vi "BRig_RT_start_v1,06.vi"() -> ()   [LabVIEW 2014]
uses:
  <vilib>/Platform/TimedLoop/XDataNode/XDataNode.xnode
  <vilib>/Platform/TimedLoop/XDataNode/nitl_modes.ctl
  <vilib>/Platform/TimedLoop/XDataNode/XDNodeRunTimeDep.lvlib
  <vilib>/Platform/TimedLoop/XDataNode/wakeup.ctl
  <vilib>/Platform/TimedLoop/XDataNode/timing_clust.ctl
  <vilib>/rvi/interface/nirviReadWriteControl/nirviReadWriteControl.xnode
  <vilib>/rvi/interface/Simulation/niFpgaSimulationCallBeginRW.vi
  <vilib>/rvi/errors/niLvFpgaAdjustHostInterfaceError.vi
  <vilib>/rvi/interface/nirviCloseFPGA/nirviCloseFPGA.xnode
  <vilib>/myRIO/Instrument Drivers/Utilities/Utilities.lvlib
  <vilib>/rvi/interface/nirviOpenFPGA/nirviOpenFPGA.xnode
  myRIO_BRig_RT__Case_Exp_stateList.ctl
  myRIO_BRig_RT__Case_NonExp_stateList.ctl
  <vilib>/WebDAVClient/Advanced/SessionHandle.ctl
  <vilib>/WebDAVClient/NI_WebDAV.lvlib
  <vilib>/Utility/file.llb/Read From Spreadsheet File (I64).vi
  <vilib>/Utility/file.llb/Write To Spreadsheet File (DBL).vi
  BRig_FPGA_v3,91__build.lvbitx
  BRig_FPGA_v3,91.vi
  <vilib>/FPGAPlugInAG/Dynamic/niLvFpga_Close_Dynamic.vi
panel:
  out "FreeReward_c_R":u16
  out "FreeReward_c_L":u16
  in  "Laser2_LED":bool
  in  "Laser1_LED":bool
  in  "lick_Rising(F)_or_Falling(T)":bool
  out "T_ExpRun_min":dbl
  out "stop_TimedLoop":bool
  out "BTPR_avg_R":dbl
  out "T2R_avg_R":dbl
  out "BTPR_avg_L":dbl
  out "T2R_avg_L":dbl
  out "BTPR_block":u16
  out "T2R_block":u16
  in  "comm_WebDAV_connect":bool
  in  "I_sendData":bool
  in  "comm_TCP_connect":bool
  out "nRewards_total":u16 caption="# Rewards in Current Block"
  out "BUR_target":u16 caption="Target Trials Per Block"
  in  "input_Threshold_reset":bool
  out "nTrial":u16
  out "allReward_R":bool
  out "allReward_L":bool
  out "Threshold":bool
  out "tLoop":dbl format="%#_2g"
  out "L_Power_l2":dbl
  out "comm_TCP":bool
  in  "get_countPerMS":bool
  out "SolenoidReward":bool
  out "L_Power_l1":dbl caption="LaserPower"
  in  "Recording":bool
  out "FPGA_count2ms":dbl=159.0
  out "error out":errorcluster
  out "cSpout":enum16{"Left", "Right"}(ring) caption="Left or Right Spout"
  out "A4":u32 caption="LickCounter_Right"
  out "A2":u32 caption="LickCounter_Left"
  out "nRewards_Right":u16 caption="# Rewards Total (Right)"
  out "nRewards_Left":u16 caption="# Rewards Total (Left)"
  out "nRewards_cur":u16 caption="# Rewards in Current Block"
  out "TpB_target":u16 caption="Target Trials Per Block"
  out "cState_NonExp":T1 caption="WarmUp State"
  out "iBlock":u16 caption="Current Block"
  out "cState":T2 caption="Experimental State"
  out "iTrial":u16 caption="Current Trial"
  in  "Data Set Prefix":string="Exp1_TM2"
  out "comm_WebDAV":bool
  in  "Host Password":string="sabalab"
  in  "Host UserName":string="Test2"
  in  "STOP_abort":bool caption="Stop LabView\n(Stops myRio and FPGA)"
  in  "STOP_endBlock":bool caption="Stop Experiment\n@ End of Block"
  in  "STOP_endTrial":bool caption="Stop Experiment\n@ End of Trial"
  in  "START":bool caption="Start Experiment"
  # "Experimental Run"
  # "Recording Rig"
  # "FPGA Conversion\n[counts per ms]"
  # "RealTime Cycle\nShould be <5ms"
  # "STOP experiment at"
  # "Exp Run Time"
  # "Reset"
  # "min"
  # "Communication with Host"
  # "Test AnalogInput Plotting"
  # "Lick Counter"
  # "Give Water?\n(Reward)"
  # "Experimental State"
  # "Left/Right"
  # "AI0               AI1"
  # "Left           Right"
  # "Direction\n(NonSpecific Licking)"
  # "Block Target"
  # "# Blocks"
  # "L          R"
  # "# Trials"
  # "# Rewards"
  # "Bad Trials\nPost Reward"
  # "Trials 2 Reward"
  # "Block"
  # "# Trials"
  # "# Rewards"
  # "Current\nBlock"
  # "WarmUp State"
  # "avg L"
  # "Total"
  # "# Rewards"
  # "# Trials"
  # "avg R"
  # "Laser Power [V]"
  # "Left           Right"
  # "FreeRewards"
  # "Laser1"
  # "Laser2"
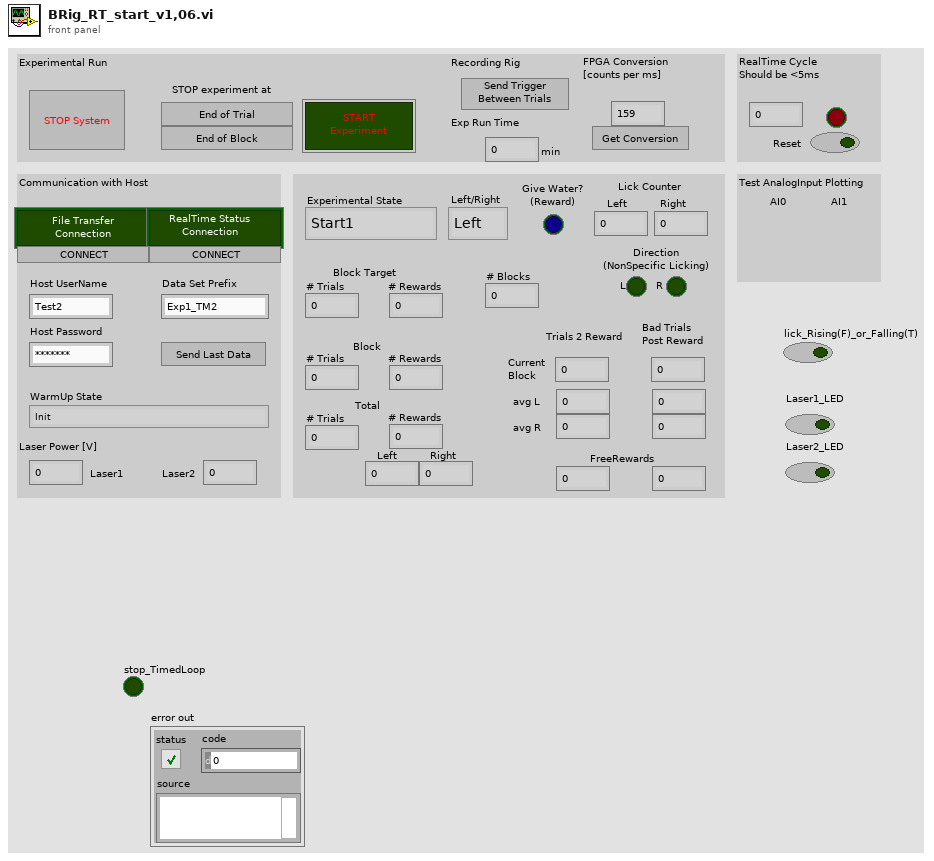
[diagram p1: front panel]
types:
  T1 = typedef "myRIO_BRig_RT__Case_NonExp_stateList.ctl" = enum16{"Init", "UploadSettings_pre", "UploadSettings_Read_dataExp", "UploadSettings_dataExp_1", "UploadSettings_dataExp_2", "UploadSettings_Read_dataLC", "UploadSettings_dataLC_1", "UploadSettings_dataLC_2", "UploadSettings_dataLC_3", "UploadSettings_dataLC_4", "UploadSettings_Read_dataMTrig", "UploadSettings_dataMTrig_1", "UploadSettings_post", "Idle_pre", "IdleEmpty", "IdleEmpty2", "IdleEmpty3", "IdleEmpty4", "Idle", "Idle_2", "Idle_3", "Idle_4", "Idle_5", "Idle_6", "Idle_post", "Cue_pre__pre", "Cue_pre", "Cue", "Cue_LED", "Cue_post", "RewardCalibration_pre", "RewardCalibration", "DispenseWater_pre__pre", "DispenseWater_pre", "DispenseWater", "DispenseWater_post", "TestConnection", "SendData", "Get_FPGA_count_per_ms", "End", "commTCP_connect"}
  T2 = typedef "myRIO_BRig_RT__Case_Exp_stateList.ctl" = enum16{"Start1", "Start2", "Start3", "saveSettings1", "saveSettings2", "saveSettings3", "saveSettings4", "saveSettings_LC_ENL_l1", "saveSettings_LC_ENL_l2", "saveSettings_LC_Cue_l1", "saveSettings_LC_Cue_l2", "saveSettings6_LC_l1_Other", "SaveSettings6_LC_l2_Other", "setSettings_Audio", "setSettings_Laser", "initBlock_pre", "initBlock", "initBlock2", "initBlock_post", "initTrial_pre", "initTrial", "initTrial2", "initTrial3", "initTrial4", "initTrial_LC_ENL1", "initTrial_LC_Cue1", "initTrial_LC_Cue1_2", "initTrial_LC_Sel", "initTrial_post", "ENL1_pre", "ENL1", "ENL1_post", "ENL1Penalty_pre", "ENL1Penalty", "ENL2_pre", "ENL2", "ENL2Penalty_pre", "ENL2Penalty", "Cue1_pre", "Cue1", "Cue1_post", "Cue1Penalty_pre", "Cue1Penalty", "Cue2_pre", "Cue2", "Cue2Penalty_pre", "Cue2Penalty", "Selection_pre", "Selection", "Select_post", "SelectReward_pre", "SelectReward", "SelectRewardPost_pre", "SelectRewardPost", "SelectWrong_pre", "SelectWrong", "SelectWrong_post", "SelectTimeout_pre", "SelectTimeout", "SelectTimeout_post", "endTrial_pre", "endTrial1", "endTrial2", "endTrial3", "endTrial_post", "endBlock_pre", "endBlock", "endBlock_post", "endExp", "commConnect", "commUpload_pre", "commUpload_dataBlock", "commUpload_dataCurrent", "commUpload_dataExp", "commUpload_dataLC", "commUpload_dataTrial", "commUpload_post", "saveData_pre", "saveData_dataBlock", "saveData_dataCurrent", "saveData_dataExp", "saveData_dataLC", "saveData_dataTrial", "saveData_post", "empty_endBlock1", "empty_endBlock2", "empty_endTrial1", "empty_endTrial2", "empty_endTrial3", "empty_endTrial4", "empty_endTrial5", "dummyState", "dummyState_endBlock", "FreeReward_pre", "FreeReward", "FreeRewardPost_pre", "FreeRewardPost"}
  T3 = enum8{"Enabled", "Disabled", "Disabled and Grayed Out"}
  T4 = typedef "NI_WebDAV.lvlib/SessionHandle.ctl" = refnum<k1>
  T5 = typedef "XDNodeRunTimeDep.lvlib/timing_clust.ctl" = cluster{"Expected End [f-1]":u64, "Actual End [f-1]":u64, "Finished Late? [f-1]":bool, "Expected End [i-1]":u64, "Actual End [i-1]":u64, "Finished Late? [i-1]":bool, "Expected Start [i]":u64, "Actual Start [i]":u64, "Expected Start [f]":u64, "Actual Start [f]":u64, "Source Name":string, "Structure Name":string, "Period":i64, "Deadline":i64, "Offset":i64, "Start":i64, "Priority":i32, "Timeout":i32, "Mode":T6, "Wakeup Reason":T7, "Error":errorcluster, "Source Type":string, "Secondary Source Type":string, "Global End Time":u64, "Global Start Time":u64, "Frame Duration":u64, "Iteration Duration":u64, "Assigned CPU":i32, "I/O Scan Engine Mode":u32}
  T6 = typedef "XDNodeRunTimeDep.lvlib/nitl_modes.ctl" = enum32{"No Change", "Process missed periods, maintain original phase", "Discard missed periods, maintain original phase", "Process missed periods, ignore original phase", "Discard missed periods, ignore original phase"}
  T7 = typedef "XDNodeRunTimeDep.lvlib/wakeup.ctl" = enum32{"Normal", "Aborted", "Asynchronous wakeup", "Timing source error", "Timed loop error", "Timeout"}
  T8 = cluster{"read mode":enum16{"polling", "blocking"}, "write mode":enum16{"polling", "blocking"}}
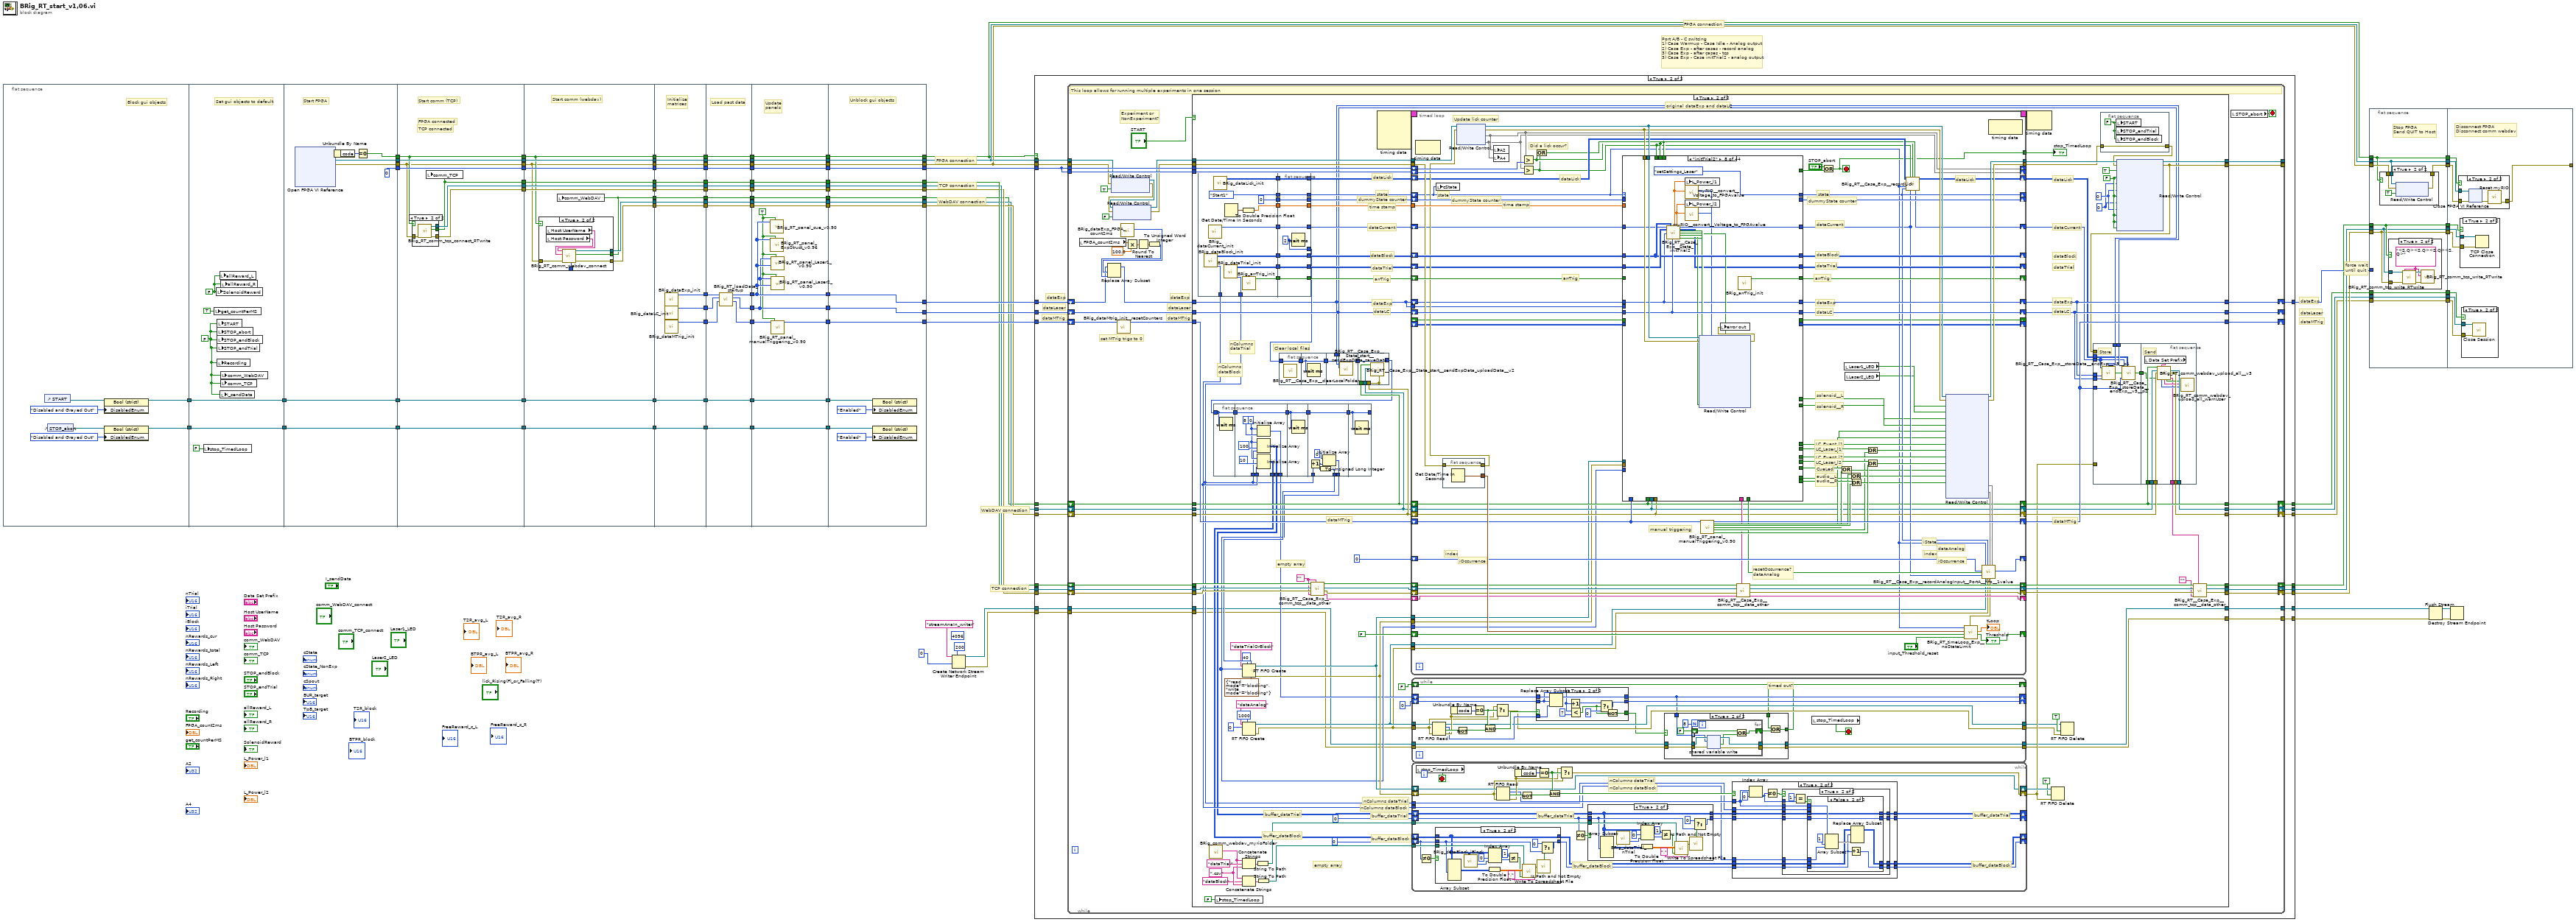
[diagram p0: block diagram]
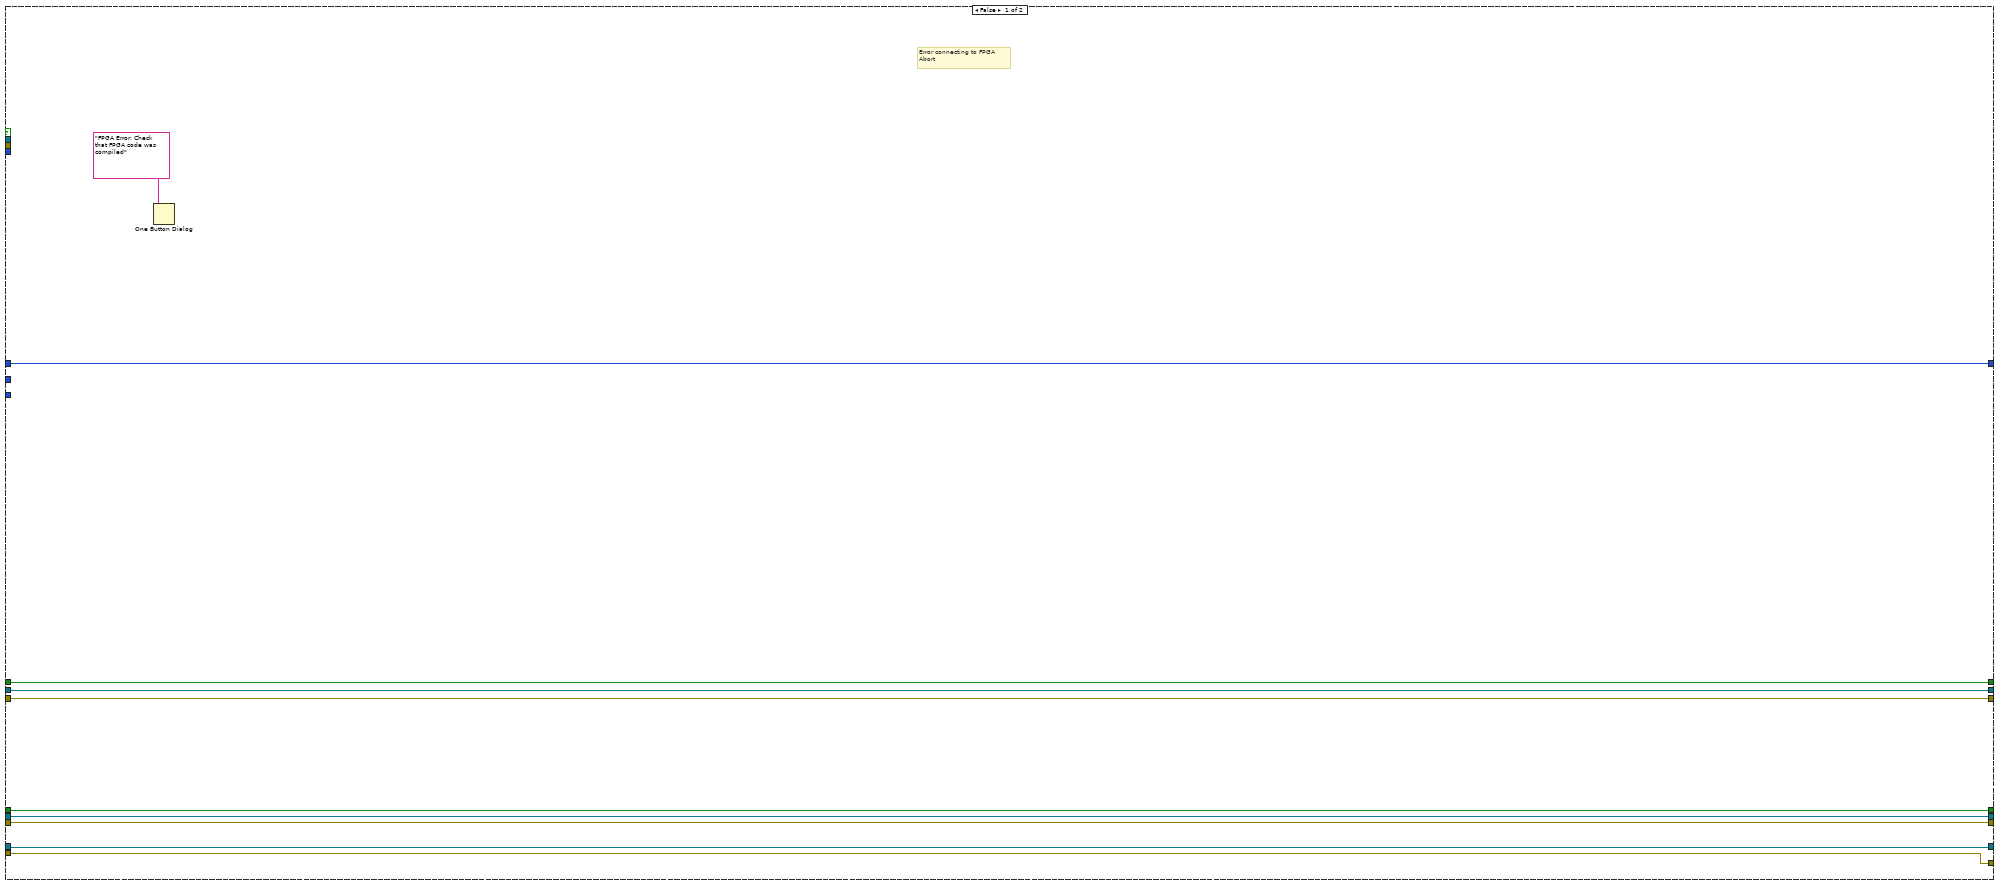
[diagram p2: hidden frame]
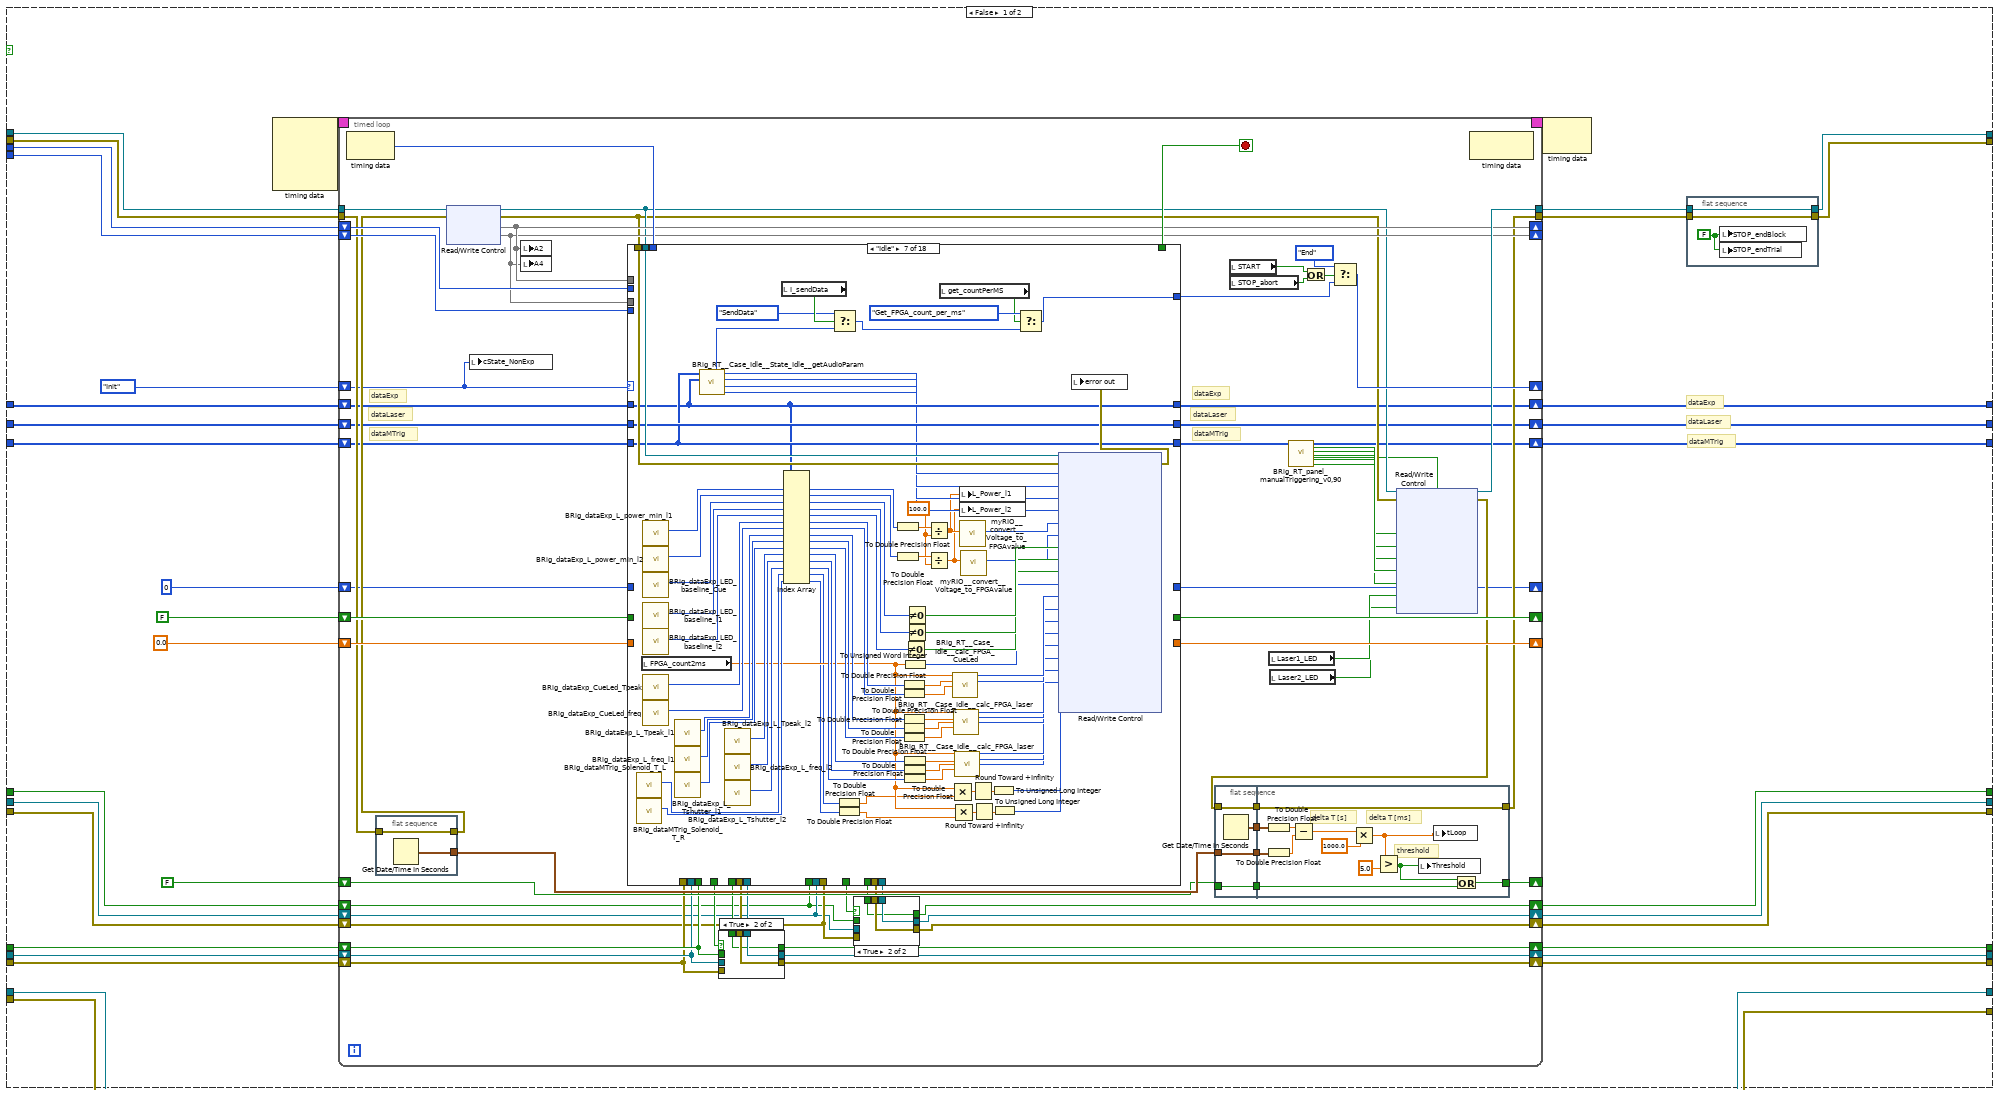
[diagram p3: hidden frame]
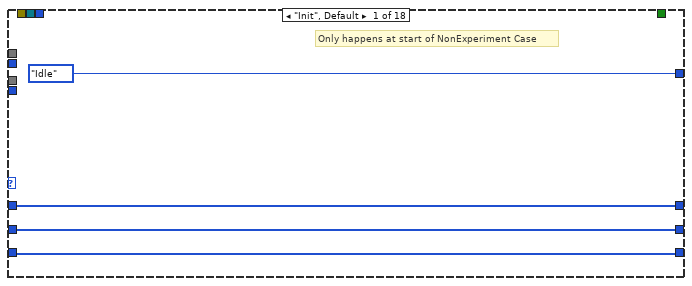
[diagram p6: hidden frame]
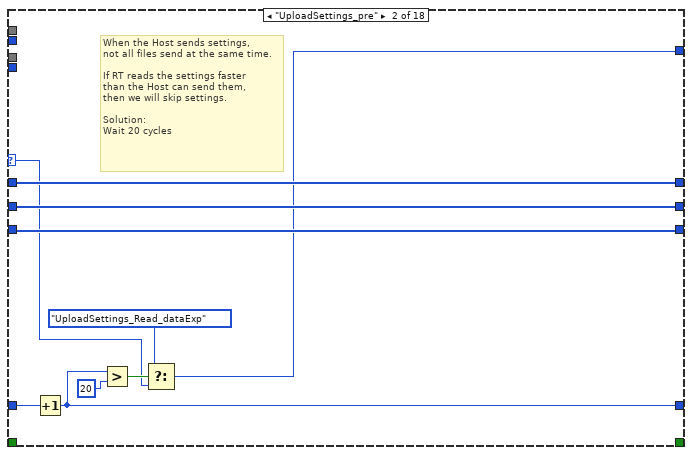
[diagram p7: hidden frame]
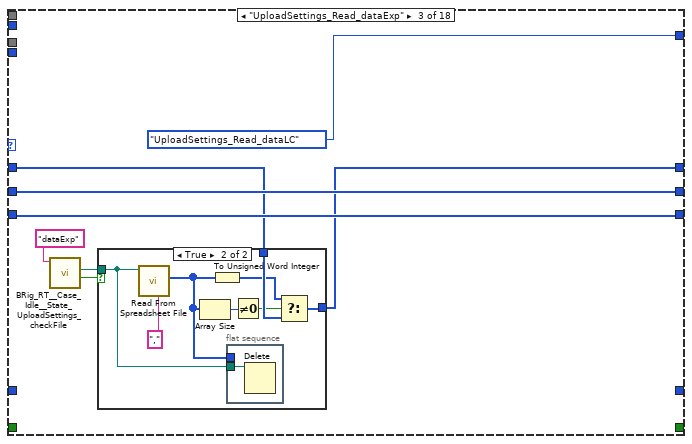
[diagram p8: hidden frame]
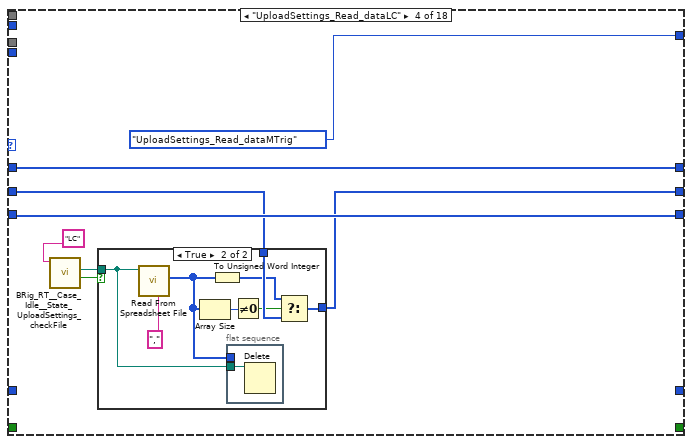
[diagram p10: hidden frame]
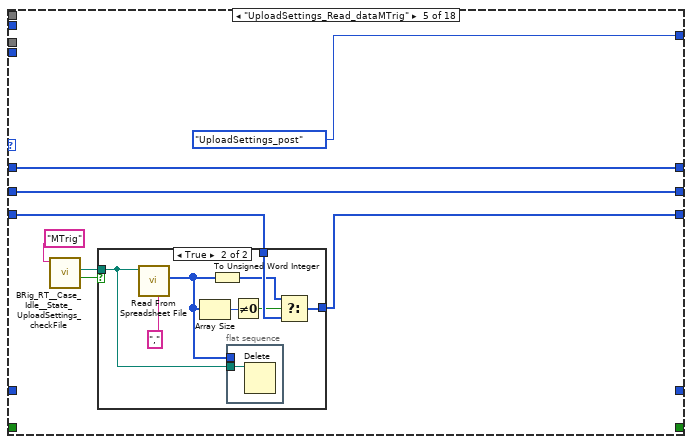
[diagram p12: hidden frame]
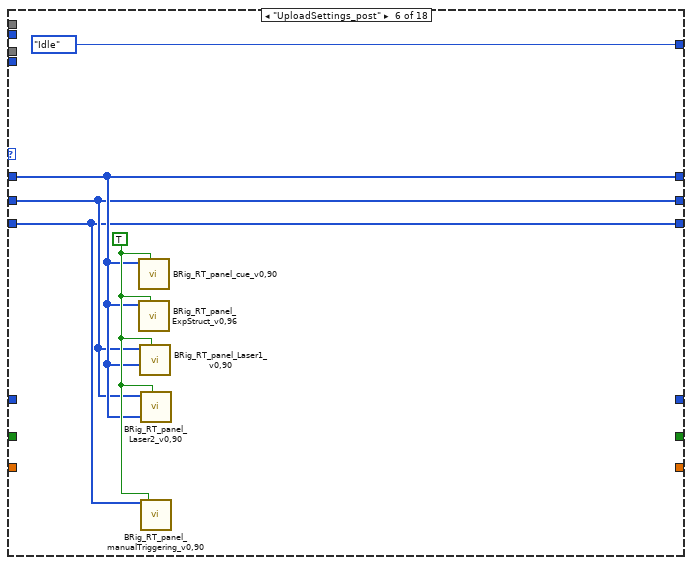
[diagram p14: hidden frame]
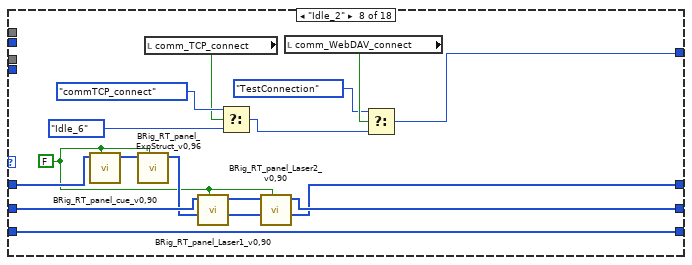
[diagram p15: hidden frame]
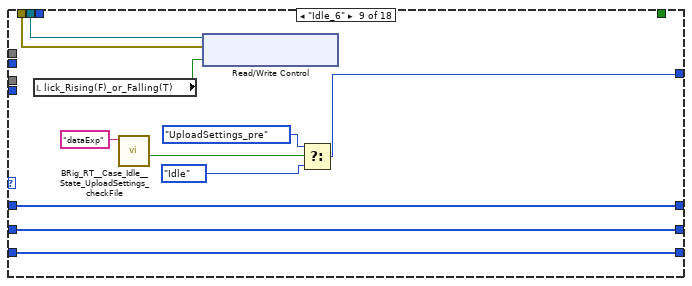
[diagram p16: hidden frame]
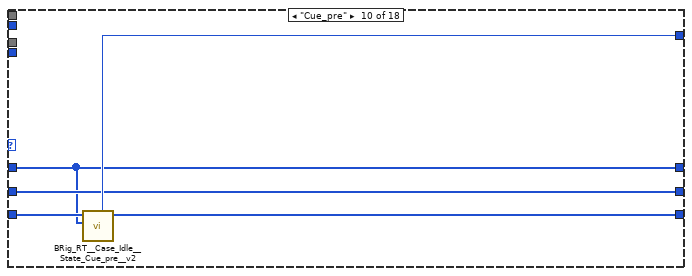
[diagram p17: hidden frame]
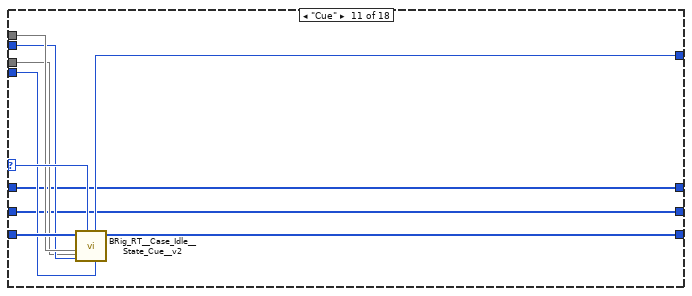
[diagram p18: hidden frame]
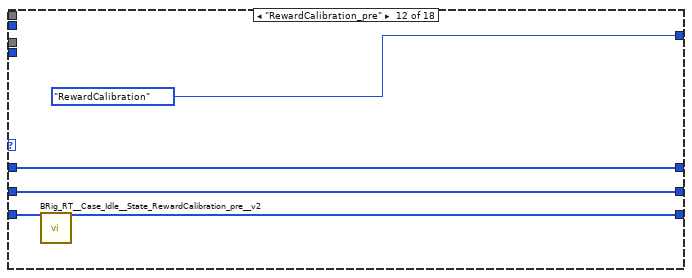
[diagram p19: hidden frame]
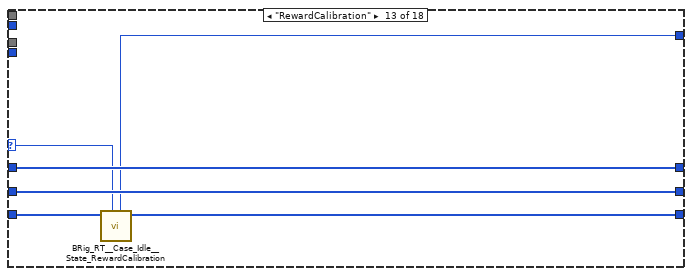
[diagram p20: hidden frame]
diagram:
  (unwired) 4096 ("reader buffer size")
  # "WebDAV connection"
  # "TCP connection"
  # "WebDAV connection"
  # "TCP connection"
  # "FPGA connection"
  # "FPGA connection"
  # "Port A/B - C switcing\n1) Case Warmup - Case Idle - Analog output\n2) Case Exp - after cases - record analog\n3) Case Exp - after cases - tcp\n3) Case Exp - Case initTrial2 - analog output"
  # "force wait\nuntil quit"
  # "dataLaser"
  # "dataExp"
  # "dataMTrig"
  n1 = flat-sequence {
    tunnel: [w116] -> w99
    tunnel: [w115] -> w95
    tunnel: [w125] -> w100
    tunnel: w99 -> [w125]
    tunnel: [w124] -> w96
    tunnel: w95 -> [w124]
    tunnel: [w131] -> w113
    tunnel: [w133] -> w112
    tunnel: [u32 0] -> w111
    tunnel: [w129] -> w110
    tunnel: [w128] -> w101
    tunnel: w100 -> [w128]
    tunnel: [w127] -> w97
    tunnel: w96 -> [w127]
    tunnel: w113 -> [w139]
    tunnel: w112 -> [w142]
    tunnel: w111 -> [w141]
    tunnel: w110 -> [w140]
    tunnel: [w139] -> w109
    tunnel: [w142] -> w108
    tunnel: [w141] -> w107
    tunnel: [w140] -> w106
    tunnel: [w134] -> w105
    tunnel: [w138] -> w104
    tunnel: [w137] -> w103
    tunnel: [w136] -> w102
    tunnel: w101 -> [w136]
    tunnel: [w135] -> w98
    tunnel: w97 -> [w135]
    tunnel: w109 -> [w153]
    tunnel: w108 -> [w161]
    tunnel: w107 -> [w160]
    tunnel: w106 -> [w154]
    tunnel: w105 -> [w159]
    tunnel: w104 -> [w158]
    tunnel: w103 -> [w157]
    tunnel: [w153] -> w66
    tunnel: [w161] -> w65
    tunnel: [w160] -> w64
    tunnel: [w154] -> w63
    tunnel: [w159] -> w62
    tunnel: [w158] -> w61
    tunnel: [w157] -> w60
    tunnel: [w156] -> w59
    tunnel: w102 -> [w156]
    tunnel: [w155] -> w58
    tunnel: w98 -> [w155]
    tunnel: [w152] -> w57
    tunnel: [w150] -> w56
    tunnel: [w151] -> w55
    tunnel: w66 -> [w186]
    tunnel: [w186] -> w54
    tunnel: w65 -> [w185]
    tunnel: [w185] -> w53
    tunnel: w64 -> [w184]
    tunnel: [w184] -> w52
    tunnel: w63 -> [w183]
    tunnel: [w183] -> w51
    tunnel: w62 -> [w182]
    tunnel: [w182] -> w50
    tunnel: w61 -> [w181]
    tunnel: [w181] -> w49
    tunnel: w60 -> [w180]
    tunnel: [w180] -> w48
    tunnel: w59 -> [w179]
    tunnel: [w179] -> w47
    tunnel: w58 -> [w178]
    tunnel: [w178] -> w46
    tunnel: w57 -> [w177]
    tunnel: [w177] -> w45
    tunnel: w56 -> [w176]
    tunnel: [w176] -> w44
    tunnel: w55 -> [w175]
    tunnel: [w175] -> w43
    tunnel: [w174] -> w42
    tunnel: [w173] -> w41
    tunnel: [w172] -> w40
    tunnel: w54 -> [w204]
    tunnel: [w204] -> w39
    tunnel: w53 -> [w203]
    tunnel: [w203] -> w37
    tunnel: w52 -> [w202]
    tunnel: [w202] -> w35
    tunnel: w51 -> [w201]
    tunnel: [w201] -> w33
    tunnel: w50 -> [w200]
    tunnel: [w200] -> w31
    tunnel: w49 -> [w199]
    tunnel: [w199] -> w29
    tunnel: w48 -> [w198]
    tunnel: [w198] -> w27
    tunnel: w47 -> [w197]
    tunnel: [w197] -> w25
    tunnel: w46 -> [w196]
    tunnel: [w196] -> w23
    tunnel: w45 -> [w195]
    tunnel: [w195] -> w21
    tunnel: w44 -> [w194]
    tunnel: [w194] -> w19
    tunnel: w43 -> [w193]
    tunnel: [w193] -> w17
    tunnel: w42 -> [w188]
    tunnel: [w187] -> w15
    tunnel: w41 -> [w190]
    tunnel: [w189] -> w13
    tunnel: w40 -> [w192]
    tunnel: [w191] -> w12
    tunnel: w39 -> [w221]
    tunnel: [w221] -> w38
    tunnel: w37 -> [w220]
    tunnel: [w220] -> w36
    tunnel: w35 -> [w219]
    tunnel: [w219] -> w34
    tunnel: w33 -> [w218]
    tunnel: [w218] -> w32
    tunnel: w31 -> [w217]
    tunnel: [w217] -> w30
    tunnel: w29 -> [w216]
    tunnel: [w216] -> w28
    tunnel: w27 -> [w215]
    tunnel: [w215] -> w26
    tunnel: w25 -> [w214]
    tunnel: [w214] -> w24
    tunnel: w23 -> [w213]
    tunnel: [w213] -> w22
    tunnel: w21 -> [w212]
    tunnel: [w212] -> w20
    tunnel: w19 -> [w211]
    tunnel: [w211] -> w18
    tunnel: w17 -> [w210]
    tunnel: [w210] -> w16
    tunnel: w15 -> [w207]
    tunnel: [w206] -> w14
    tunnel: w13 -> [w208]
    tunnel: w12 -> [w209]
    tunnel: [w209] -> w11
    tunnel: [w208] -> w10
    tunnel: [w228] -> w76
    tunnel: [w229] -> w77
    tunnel: [w230] -> w78
    tunnel: [w235] -> w82
    tunnel: [w236] -> w114
    tunnel: [w237] -> w89
    tunnel: [w238] -> w88
    tunnel: w38 -> [w238]
    tunnel: w36 -> [w237]
    tunnel: w34 -> [w236]
    tunnel: w32 -> [w235]
    tunnel: w30 -> [w230]
    tunnel: w28 -> [w229]
    tunnel: w26 -> [w228]
    tunnel: w24 -> [w232]
    tunnel: w22 -> [w231]
    tunnel: w20 -> [w226]
    tunnel: w18 -> [w227]
    tunnel: w16 -> [w225]
    tunnel: [w227] -> w70
    tunnel: [w226] -> w71
    tunnel: [w225] -> w72
    tunnel: [w222] -> w85
    tunnel: [w223] -> w84
    tunnel: [w224] -> w83
    tunnel: w14 -> [w224]
    tunnel: w11 -> [w222]
    tunnel: w10 -> [w223]
    frame #0 {
      # "Block gui objects"
      n2 = control-ref of="START"() -> (w120:refnum<vi>)
      n3 = control-ref of="STOP_abort"() -> (w117:refnum<vi>)
      n4 = property class="Bool (strict)"(reference=w120, "DisabledEnum"=T3."Disabled and Grayed Out" ("Disabled")) -> (reference out=w116:refnum<vi>)  [unwired: 1 in, 1 out]
      n5 = property class="Bool (strict)"(reference=w117, "DisabledEnum"=T3."Disabled and Grayed Out" ("Disabled")) -> (reference out=w115:refnum<vi>)  [unwired: 1 in, 1 out]
    }
    frame #1 {
      w122 = FALSE ("SolenoidReward")
      w123 = FALSE
      # "Set gui objects to default"
      n6 = local write "stop_TimedLoop"(FALSE ("stop_TimedLoop")) -> ()
      n7 = local write "get_countPerMS"(TRUE ("get_countPerMS")) -> ()
      n8 = local write "SolenoidReward"(w122) -> ()
      n9 = local write "START"(w123) -> ()
      n10 = local write "STOP_abort"(w123) -> ()
      n11 = local write "STOP_endBlock"(w123) -> ()
      n12 = local write "STOP_endTrial"(w123) -> ()
      n13 = local write "Recording"(w123) -> ()
      n14 = local write "allReward_L"(w122) -> ()
      n15 = local write "I_sendData"(w123) -> ()
      n16 = local write "comm_WebDAV"(w123) -> ()
      n17 = local write "comm_TCP"(w123) -> ()
      n18 = local write "allReward_R"(w122) -> ()
    }
    frame #2 {
      # "Start FPGA"
      n19 = xnode "Open FPGA VI Reference"() -> ("FPGA VI Reference Out"=w133:refnum<k20>, "error out"=w131:errorcluster)  [unwired: 2 in]
      n20 = Unbundle By Name(w131) -> ("code"=w130:i32)
      n21 = Equal To 0?(x=w130) -> (x = 0?=w129:bool)
    }
    frame #3 {
      # "TCP connected"
      # "Start comm (TCP)"
      # "FPGA connected"
      n22 = case shown="True" w140 {
        selector: w140 -> [w143 _]
        tunnel: w139 -> [w145 w149]
        tunnel: [refnum<k5> refnum ("output_hTCP") w148] -> w138
        tunnel: [w143 w147] -> w134
        tunnel: [w145 w146] -> w137
        frame False {
        }
        frame True {
          n23 = call "BRig_RT_comm_tcp_connect_RTwrite.vi"("input_error"=w149) -> ("output_error"=w146:errorcluster, "output_connected"=w147:bool, "output_hTCP"=w148:refnum<k5>)  [unwired: 8 in]
        }
      }
      n24 = local write "comm_TCP"(w134) -> ()
    }
    frame #4 {
      # "Start comm (webdav)"
      n25 = case shown="True" w154 {
        selector: w154 -> [w163 _]
        tunnel: [w162 w169] -> w152
        tunnel: [w163 w168] -> w150
        tunnel: w153 -> [w164 w167]
        tunnel: [w164 w166] -> w151
        tunnel: [_ w165] -> _
        frame False {
          w162 = T4 refnum items=["Session NI_WebDAV"] ("output_hSession")
        }
        frame True {
          n26 = local read "Host UserName"() -> (w170:string)
          n27 = local read "Host Password"() -> (w171:string)
          n28 = call "BRig_RT_comm_webdav_connect.vi"("input_error"=w167, "input_password"=w171, "input_username"=w170) -> ("output_error"=w166:errorcluster, "output_Iconnected"=w168:bool, "output_hSession"=w169:T4, "output_code"=w165:u8)  [unwired: 5 in]
        }
      }
      n29 = local write "comm_WebDAV"(w150) -> ()
    }
    frame #5 {
      # "Initialize\nmatrices"
      n30 = call "BRig_dataExp_init.vi"() -> ("output_dataExp"=w172:u16[])  [unwired: 11 in]
      n31 = call "BRig_dataLC_init.vi"() -> ("output_dataLC"=w173:u16[])  [unwired: 11 in]
      n32 = call "BRig_dataMTrig_init.vi"() -> ("output_dataMTrig"=w174:u16[])  [unwired: 5 in]
    }
    frame #6 {
      # "Load past data"
      n33 = call "BRig_RT_loadData_startup.vi"("input_dataMTrig"=w188, "input_dataLC"=w190, "input_dataExp"=w192) -> ("output_dataMTrig"=w187:u16[], "output_dataLC"=w189:u16[], "output_dataExp"=w191:u16[])  [unwired: 6 in]
    }
    frame #7 {
      w205 = TRUE ("input_setValues")
      # "Update\npanels"
      n34 = call "BRig_RT_panel_cue_v0,90.vi"("input_setValues"=w205, "input_dataExp"=w209) -> ()  [unwired: 9 in, 1 out]
      n35 = call "BRig_RT_panel_ExpStruct_v0,96.vi"("input_setValues"=w205, "input_dataExp"=w209) -> ()  [unwired: 9 in, 1 out]
      n36 = call "BRig_RT_panel_Laser1_v0,90.vi"("input_setValues"=w205, "input_dataExp"=w209, "input_dataLC"=w208) -> ()  [unwired: 7 in, 2 out]
      n37 = call "BRig_RT_panel_Laser2_v0,90.vi"("input_setValues"=w205, "input_dataExp"=w209, "input_dataLC"=w208) -> ()  [unwired: 7 in, 2 out]
      n38 = call "BRig_RT_panel_manualTriggering_v0,90.vi"("input_dataMTrig"=w207, "input_setValues"=w205) -> ("output_dataMTrig"=w206:u16[])  [unwired: 10 in, 7 out]
    }
    frame #8 {
      # "Unblock gui objects"
      n39 = property class="Bool (strict)"(reference=w232, "DisabledEnum"=T3."Enabled" ("Disabled")) -> ()  [unwired: 1 in, 2 out]
      n40 = property class="Bool (strict)"(reference=w231, "DisabledEnum"=T3."Enabled" ("Disabled")) -> ()  [unwired: 1 in, 2 out]
    }
  }
  n41 = Create Network Stream Writer Endpoint(7:200 ("reader buffer size"), 9:u16 0 ("element"), 11:"streamAnaIn_writer" ("reader name")) -> (0:w2:errorcluster, 3:w3:refnum<k21>)  [unwired: 4 in]
  n42 = case shown="True" w82 {
    tunnel: w114 -> [_ w271]
    tunnel: w89 -> [_ w270]
    tunnel: w88 -> [_ w269]
    tunnel: [w248 w268] -> w86
    tunnel: w85 -> [w248 w267]
    tunnel: w84 -> [_ w266]
    tunnel: w83 -> [_ w265]
    tunnel: w78 -> [w247 w264]
    tunnel: w77 -> [w246 w263]
    tunnel: w76 -> [w245 w262]
    tunnel: [w247 w261] -> w75
    tunnel: [w246 w260] -> w74
    tunnel: [w245 w259] -> w73
    tunnel: w72 -> [w244 w258]
    tunnel: w71 -> [w243 w257]
    tunnel: w70 -> [w242 w256]
    tunnel: [w244 w255] -> w69
    tunnel: [w243 w254] -> w68
    tunnel: [w242 w253] -> w67
    tunnel: [w241 w252] -> w7
    tunnel: [w240 w251] -> w6
    tunnel: w3 -> [w241 w250]
    tunnel: w2 -> [w240 w249]
    frame False {
      # "Error connecting to FPGA\nAbort"
      n43 = One Button Dialog(message="FPGA Error: Check that FPGA code was compiled") -> ()  [unwired: 1 in, 1 out]
    }
    frame True {
      # "dataExp"
      # "dataLaser"
      # "dataMTrig"
      n44 = while {
        tunnel: w270 -> [w305]
        tunnel: w269 -> [w310]
        tunnel: w271 -> [w313]
        tunnel: w271 -> [w312]
        tunnel: [w303] -> _
        tunnel: [w302] -> _
        shift-right: [w301] -> _
        shift-left: w265 -> [w297]
        shift-right: [w299] -> _
        shift-left: w266 -> [w300]
        shift-right: [w298] -> w268
        shift-left: w267 -> [w277]
        shift-right: [w292] -> w261
        shift-left: w264 -> [w295]
        shift-right: [w291] -> w260
        shift-left: w263 -> [w294]
        shift-right: [w290] -> w259
        shift-left: w262 -> [w293]
        shift-right: [w286] -> w255
        shift-left: w258 -> [w289]
        shift-right: [w285] -> w254
        shift-left: w257 -> [w288]
        shift-right: [w284] -> w253
        shift-left: w256 -> [w287]
        tunnel: [w275] -> w252
        tunnel: [w274] -> w251
        tunnel: w250 -> [w273]
        tunnel: w249 -> [w272]
        stop <- w311 stop-if-true
        # "set MTrig trigs to 0"
        # "dataExp"
        # "dataLaser"
        # "dataMTrig"
        # "Experiment or\nNonExperiment?"
        # "This loop allows for running multiple experiments in one session"
        n45 = local read "FPGA_count2ms"() -> (w281:dbl)
        n46 = xnode "Read/Write Control"("FPGA VI Reference In"=w305, "error in"=w310, "Counts_Reset"=TRUE) -> ("FPGA VI Reference Out"=w307:refnum<k20>, "error out"=w308:errorcluster)
        n47 = xnode "Read/Write Control"("FPGA VI Reference In"=w307, "error in"=w308, "Counts_Reset"=FALSE) -> ("FPGA VI Reference Out"=w304:refnum<k20>, "error out"=w306:errorcluster)
        n48 = call "BRig_dataMtrig_init__resetCounters.vi"("input_dataMTrig"=w297) -> ("output_dataMTrig"=w296:u16[])  [unwired: 10 in]
        n49 = call "BRig_dataExp_FPGA_count2ms.vi"() -> ("output_FPGA_count2ms"=w282:i32)  [unwired: 11 in]
        n50 = Multiply(x=w281, y=100.0) -> (x*y=w279:dbl)
        n51 = Round To Nearest(number=w279) -> (nearest integer value=w278:dbl)
        n52 = To Unsigned Word Integer(number=w278) -> (unsigned 16bit integer=w283:u16)
        n53 = Replace Array Subset(array=w277, new element=w283, index=w282) -> (w276:u16[])
        n54 = case shown="True" "START" {
          tunnel: w313 -> [w347 w910]
          tunnel: w312 -> [w346 w909]
          tunnel: w306 -> [w344 w898]
          tunnel: w304 -> [w345 w899]
          tunnel: [w342 w907] -> w303
          tunnel: [w340 w876] -> w302
          tunnel: w296 -> [w336 w896]
          tunnel: [w335 w882] -> w301
          tunnel: w300 -> [w334 w846]
          tunnel: w276 -> [w333 w797]
          tunnel: [w332 w881] -> w299
          tunnel: [w331 w880] -> w298
          tunnel: w295 -> [w330 w890]
          tunnel: w294 -> [w329 w889]
          tunnel: w293 -> [w328 w888]
          tunnel: [w327 w865] -> w292
          tunnel: [w326 w864] -> w291
          tunnel: [w325 w863] -> w290
          tunnel: w289 -> [w324 w845]
          tunnel: w288 -> [w323 w844]
          tunnel: w287 -> [w322 w843]
          tunnel: [w321 w872] -> w286
          tunnel: [w320 w871] -> w285
          tunnel: [w319 w873] -> w284
          tunnel: w273 -> [w317 w802]
          tunnel: w272 -> [w316 w801]
          tunnel: [w317 w800] -> w275
          tunnel: [w316 w799] -> w274
          frame False {
            # "dataExp"
            # "dataLaser"
            # "dataMTrig"
            n55 = node-c288() -> (w350:T5)  [unwired: 4 in]
            n56 = timed-loop {
              timing: w350 -> [_]
              timing-out: [_] -> w349
              shift-right: [w414] -> _
              shift-left: myRIO_BRig_RT__Case_NonExp_stateList."Init" ("Enum") -> [w383]
              shift-right: [w412] -> _
              shift-left: w347 -> [w413]
              shift-right: [w410] -> _
              shift-left: w346 -> [w411]
              tunnel: [w420] -> w343
              tunnel: [w396] -> w341
              tunnel: w344 -> [w403]
              tunnel: w345 -> [w421]
              shift-right: [w406] -> _
              shift-left: FALSE -> [w407]
              shift-right: [w404] -> _
              shift-left: 0.0 -> [w405]
              shift-right: [w393] -> _
              shift-left: FALSE -> [w394]
              shift-right: [w392] -> w335
              shift-left: w336 -> [w384]
              shift-right: [w378] -> w331
              shift-left: w333 -> [w381]
              shift-right: [w379] -> w332
              shift-left: w334 -> [w380]
              shift-right: [w377] -> w327
              shift-left: w330 -> [w373]
              shift-right: [w376] -> w326
              shift-left: w329 -> [w372]
              shift-right: [w375] -> w325
              shift-left: w328 -> [w371]
              shift-right: [w361] -> w321
              shift-left: w324 -> [w367]
              shift-right: [w362] -> w320
              shift-left: w323 -> [w366]
              shift-right: [w363] -> w319
              shift-left: w322 -> [w365]
              shift-right: [w356] -> _
              shift-left: u16 0 ("y") -> [w357]
              stop <- w423 stop-if-true
              # "dataExp"
              # "dataLaser"
              # "dataExp"
              # "dataLaser"
              # "dataMTrig"
              # "dataMTrig"
              n57 = node-c288() -> (w422:i64)  [unwired: 1 in]
              n58 = flat-sequence {
                tunnel: w403 -> [w452]
                tunnel: [w453] -> w395
                tunnel: [w452] -> w402
                frame #0 {
                  n59 = Get Date/Time In Seconds() -> (seconds since 1Jan1904=w453:timestamp)
                }
              }
              n60 = xnode "Read/Write Control"("FPGA VI Reference In"=w421, "error in"=w402) -> ("FPGA VI Reference Out"=w409:refnum<k20>, "error out"=w408:errorcluster, "A2_LickL"=w412, "A4_LickR"=w410)
              n61 = local write "cState_NonExp"(w383) -> ()
              n62 = local write "A2"(w412) -> ()
              n63 = local write "A4"(w410) -> ()
              n64 = case shown="\"Idle\"" w383 {
                selector: w383 -> [_ w460 _ _ _ _ _ _ _ _ w651 _ w659 _ _ w703 w746 w752]
                tunnel: [myRIO_BRig_RT__Case_NonExp_stateList."Idle" ("Enum") w461 myRIO_BRig_RT__Case_NonExp_stateList."UploadSettings_Read_dataLC" ("t") myRIO_BRig_RT__Case_NonExp_stateList."UploadSettings_Read_dataMTrig" ("t") myRIO_BRig_RT__Case_NonExp_stateList."UploadSettings_post" ("t") myRIO_BRig_RT__Case_NonExp_stateList."Idle" ("t") w544 w610 w634 w640 w649 myRIO_BRig_RT__Case_NonExp_stateList."RewardCalibration" ("Enum") w658 myRIO_BRig_RT__Case_NonExp_stateList."Idle" ("Enum") myRIO_BRig_RT__Case_NonExp_stateList."Idle" ("Enum") w702 w746 w753] -> w415
                tunnel: [w456 w467 w475 w493 w507 w522 w556 w626 w632 w641 w650 w653 w660 w674 w686 w712 w744 w761] -> w382
                tunnel: [_ _ _ _ _ _ _ _ _ _ _ _ _ _ _ _ TRUE _] -> w423
                tunnel: w384 -> [w456 w467 w475 w493 w504 w522 w556 w626 w632 w642 w652 w654 w661 w674 w686 w712 w744 w761]
                tunnel: w422 -> [_ _ _ _ _ _ _ _ _ _ _ _ _ _ _ _ _ _]
                tunnel: w413 -> [_ _ _ _ _ _ _ _ _ _ w647 _ _ _ _ _ _ _]
                tunnel: w412 -> [_ _ _ _ _ _ _ _ _ _ w648 _ _ _ _ _ _ _]
                tunnel: w411 -> [_ _ _ _ _ _ _ _ _ _ w645 _ _ _ _ _ _ _]
                tunnel: w410 -> [_ _ _ _ _ _ _ _ _ _ w646 _ _ _ _ _ _ _]
                tunnel: w409 -> [_ _ _ _ _ _ w609 _ w629 _ _ _ _ _ _ w707 _ _]
                tunnel: w408 -> [_ _ _ _ _ _ w608 _ w628 _ _ _ _ _ _ w706 _ _]
                tunnel: w407 -> [_ _ _ _ _ _ _ _ _ _ _ _ _ _ _ w711 _ _]
                tunnel: [_ _ _ _ _ _ _ _ _ _ _ _ _ _ _ TRUE _ _] -> w406
                tunnel: w405 -> [_ _ _ _ _ _ _ _ _ _ _ _ _ _ _ w709 _ _]
                tunnel: [_ _ _ _ _ _ _ _ _ _ _ _ _ _ _ w708 _ _] -> w404
                tunnel: w381 -> [w454 w465 w470 w492 w511 w524 w555 w624 w630 w638 w643 w656 w662 w671 w683 w699 w742 w759]
                tunnel: w380 -> [w455 w466 w474 w486 w508 w523 w557 w623 w631 w639 w644 w655 w663 w672 w684 w700 w743 w760]
                tunnel: [w455 w466 w474 w489 w508 w523 w557 w619 w631 w639 w644 w655 w663 w672 w684 w700 w743 w760] -> w379
                tunnel: [w454 w465 w469 w492 w511 w524 w555 w616 w630 w638 w643 w656 w662 w671 w683 w699 w742 w759] -> w378
                tunnel: [_ _ _ _ _ _ _ _ _ _ _ _ _ _ _ _ _ TRUE] -> w374
                tunnel: w373 -> [_ _ _ _ _ _ _ _ _ _ _ _ _ _ w677 _ _ w758]
                tunnel: w372 -> [_ _ _ _ _ _ _ _ _ _ _ _ _ _ w679 _ _ w754]
                tunnel: w371 -> [_ _ _ _ _ _ _ _ _ _ _ _ _ _ w678 _ _ w757]
                tunnel: [_ _ _ _ _ _ _ _ _ _ _ _ _ _ _ _ _ w756] -> w370
                tunnel: [_ _ _ _ _ _ _ _ _ _ _ _ _ _ _ _ _ w755] -> w369
                tunnel: [_ _ _ _ _ _ _ _ _ _ _ _ _ _ _ _ _ w747] -> w368
                tunnel: w365 -> [_ _ _ _ _ _ _ _ _ _ _ _ _ _ w676 _ _ _]
                tunnel: w366 -> [_ _ _ _ _ _ _ _ _ _ _ _ _ _ w682 _ _ _]
                tunnel: w367 -> [_ _ _ _ _ _ _ _ _ _ _ _ _ w664 w681 _ _ _]
                tunnel: [_ _ _ _ _ _ _ _ _ _ _ _ _ TRUE _ _ _ _] -> w364
                tunnel: [_ _ _ _ _ _ _ _ _ _ _ _ _ w666 _ _ _ _] -> w360
                tunnel: [_ _ _ _ _ _ _ _ _ _ _ _ _ w664 _ _ _ _] -> w359
                tunnel: [_ _ _ _ _ _ _ _ _ _ _ _ _ w665 _ _ _ _] -> w358
                tunnel: w357 -> [_ w459 _ _ _ _ _ _ _ _ _ _ _ _ _ _ _ _]
                tunnel: [_ w458 _ _ _ _ _ _ _ _ _ _ _ _ _ _ _ _] -> w356
                frame "Init", Default {
                  # "Only happens at start of NonExperiment Case"
                }
                frame "UploadSettings_pre" {
                  # "When the Host sends settings,\nnot all files send at the same time.\n\nIf RT reads the settings faster\nthan the Host can send them,\nthen we will skip settings.\n\nSolution:\nWait 20 cycles"
                  n65 = Increment(x=w459) -> (x+1=w458:u16)
                  n66 = Greater?(x=w458, y=u16 20) -> (0:w463:bool)
                  n67 = Select(t=myRIO_BRig_RT__Case_NonExp_stateList."UploadSettings_Read_dataExp", s=w463, f=w460) -> (s? t:f=w461:T1)
                }
                frame "UploadSettings_Read_dataExp" {
                  n68 = call "BRig_RT__Case_Idle__State_UploadSettings_checkFile.vi"("input_dataName"="dataExp") -> ("output_Iexist"=w472:bool, "output_dataPath"=w471:path)  [unwired: 9 in]
                  n69 = case shown="True" w472 {
                    tunnel: w471 -> [_ w478]
                    tunnel: w470 -> [w476 w482]
                    tunnel: [w476 w480] -> w469
                    frame False {
                    }
                    frame True {
                      n70 = call-poly <vilib>:"Read From Spreadsheet File.vi"("delimiter (\\t)"="," ("delimiter (\\t)"), "file path (dialog if empty)"=w478) -> ("first row"=w477:i64[])  [unwired: 5 in, 4 out]
                      n71 = Array Size(array=w477) -> (size(s)=w483:i32)
                      n72 = To Unsigned Word Integer(number=w477) -> (unsigned 16bit integer=w481:u16[])
                      n73 = flat-sequence {
                        tunnel: w478 -> [w485]
                        tunnel: w477 -> [_]
                        frame #0 {
                          n74 = Delete(path (use dialog)=w485) -> ()  [unwired: 4 in, 3 out]
                        }
                      }
                      n75 = Not Equal To 0?(x=w483) -> (x != 0?=w479:bool)
                      n76 = Select(t=w481, s=w479, f=w482) -> (s? t:f=w480:u16[])
                    }
                  }
                }
                frame "UploadSettings_Read_dataLC" {
                  n77 = call "BRig_RT__Case_Idle__State_UploadSettings_checkFile.vi"("input_dataName"="LC") -> ("output_Iexist"=w487:bool, "output_dataPath"=w488:path)  [unwired: 9 in]
                  n78 = case shown="True" w487 {
                    tunnel: w488 -> [_ w496]
                    tunnel: w486 -> [w494 w500]
                    tunnel: [w494 w498] -> w489
                    frame False {
                    }
                    frame True {
                      n79 = call-poly <vilib>:"Read From Spreadsheet File.vi"("delimiter (\\t)"="," ("delimiter (\\t)"), "file path (dialog if empty)"=w496) -> ("first row"=w495:i64[])  [unwired: 5 in, 4 out]
                      n80 = Array Size(array=w495) -> (size(s)=w501:i32)
                      n81 = To Unsigned Word Integer(number=w495) -> (unsigned 16bit integer=w499:u16[])
                      n82 = flat-sequence {
                        tunnel: w496 -> [w503]
                        tunnel: w495 -> [_]
                        frame #0 {
                          n83 = Delete(path (use dialog)=w503) -> ()  [unwired: 4 in, 3 out]
                        }
                      }
                      n84 = Not Equal To 0?(x=w501) -> (x != 0?=w497:bool)
                      n85 = Select(t=w499, s=w497, f=w500) -> (s? t:f=w498:u16[])
                    }
                  }
                }
                frame "UploadSettings_Read_dataMTrig" {
                  n86 = call "BRig_RT__Case_Idle__State_UploadSettings_checkFile.vi"("input_dataName"="MTrig") -> ("output_Iexist"=w505:bool, "output_dataPath"=w506:path)  [unwired: 9 in]
                  n87 = case shown="True" w505 {
                    tunnel: w506 -> [_ w514]
                    tunnel: w504 -> [w512 w518]
                    tunnel: [w512 w516] -> w507
                    frame False {
                    }
                    frame True {
                      n88 = call-poly <vilib>:"Read From Spreadsheet File.vi"("delimiter (\\t)"="," ("delimiter (\\t)"), "file path (dialog if empty)"=w514) -> ("first row"=w513:i64[])  [unwired: 5 in, 4 out]
                      n89 = Array Size(array=w513) -> (size(s)=w519:i32)
                      n90 = To Unsigned Word Integer(number=w513) -> (unsigned 16bit integer=w517:u16[])
                      n91 = flat-sequence {
                        tunnel: w514 -> [w521]
                        tunnel: w513 -> [_]
                        frame #0 {
                          n92 = Delete(path (use dialog)=w521) -> ()  [unwired: 4 in, 3 out]
                        }
                      }
                      n93 = Not Equal To 0?(x=w519) -> (x != 0?=w515:bool)
                      n94 = Select(t=w517, s=w515, f=w518) -> (s? t:f=w516:u16[])
                    }
                  }
                }
                frame "UploadSettings_post" {
                  w525 = TRUE ("input_setValues")
                  n95 = call "BRig_RT_panel_cue_v0,90.vi"("input_setValues"=w525, "input_dataExp"=w524) -> ()  [unwired: 9 in, 1 out]
                  n96 = call "BRig_RT_panel_ExpStruct_v0,96.vi"("input_setValues"=w525, "input_dataExp"=w524) -> ()  [unwired: 9 in, 1 out]
                  n97 = call "BRig_RT_panel_Laser1_v0,90.vi"("input_setValues"=w525, "input_dataExp"=w524, "input_dataLC"=w523) -> ()  [unwired: 7 in, 2 out]
                  n98 = call "BRig_RT_panel_Laser2_v0,90.vi"("input_setValues"=w525, "input_dataExp"=w524, "input_dataLC"=w523) -> ()  [unwired: 7 in, 2 out]
                  n99 = call "BRig_RT_panel_manualTriggering_v0,90.vi"("input_dataMTrig"=w522, "input_setValues"=w525) -> ()  [unwired: 10 in, 8 out]
                }
                frame "Idle" {
                  w601 = 100.0 ("y")
                  n100 = call "BRig_dataMTrig_Solenoid_T_L.vi"() -> ("output_Solenoid_T_L"=w539:i32)  [unwired: 11 in]
                  n101 = call "BRig_dataMTrig_Solenoid_T_R.vi"() -> ("output_Solenoid_T_R"=w538:i32)  [unwired: 11 in]
                  n102 = local read "FPGA_count2ms"() -> (w537:dbl)
                  n103 = call "BRig_dataExp_L_power_min_l1.vi"() -> ("output_L_power_min_l1"=w606:i32)  [unwired: 11 in]
                  n104 = call "BRig_dataExp_L_power_min_l2.vi"() -> ("output_L_power_min_l2"=w605:i32)  [unwired: 11 in]
                  n105 = call "BRig_dataExp_LED_baseline_Cue.vi"() -> ("output_LED_baseline_Cue"=w599:i32)  [unwired: 11 in]
                  n106 = call "BRig_dataExp_LED_baseline_l1.vi"() -> ("output_LED_baseline_l1"=w598:i32)  [unwired: 11 in]
                  n107 = call "BRig_dataExp_LED_baseline_l2.vi"() -> ("output_LED_baseline_l2"=w597:i32)  [unwired: 11 in]
                  n108 = call "BRig_dataExp_CueLed_Tpeak.vi"() -> ("output_CueLed_Tpeak"=w589:i32)  [unwired: 11 in]
                  n109 = call "BRig_dataExp_CueLed_freq.vi"() -> ("output_CueLed_Freq"=w588:i32)  [unwired: 11 in]
                  n110 = call "BRig_dataExp_L_Tpeak_l1.vi"() -> ("output_L_Tpeak_l1"=w581:i32)  [unwired: 11 in]
                  n111 = call "BRig_dataExp_L_freq_l1.vi"() -> ("output_L_freq_l1"=w580:i32)  [unwired: 11 in]
                  n112 = call "BRig_dataExp_L_Tshutter_l1.vi"() -> ("output_L_Tshutter_l1"=w579:i32)  [unwired: 11 in]
                  n113 = call "BRig_RT__Case_Idle__State_Idle__getAudioParam.vi"("input_dataExp"=w555, "input_dataMTrig"=w556) -> ("output_Audio_freq_R"=w551:u8, "output_Audio_amp_R"=w552:u16, "output_Audio_freq_L"=w553:u8, "output_Audio_amp_L"=w554:u16, "output_state"=w550:T1)  [unwired: 5 in]
                  n114 = call "BRig_dataExp_L_Tpeak_l2.vi"() -> ("output_L_Tpeak_l2"=w563:i32)  [unwired: 11 in]
                  n115 = call "BRig_dataExp_L_freq_l2.vi"() -> ("output_L_freq_l2"=w562:i32)  [unwired: 11 in]
                  n116 = call "BRig_dataExp_L_Tshutter_l2.vi"() -> ("output_L_Tshutter_l2"=w561:i32)  [unwired: 11 in]
                  n117 = local read "I_sendData"() -> (w549:bool)
                  n118 = Index Array(array=w555, index #1=w606, index #2=w605, index #3=w599, index #4=w598, index #5=w597, index #6=w589, index #7=w588, index #8=w581, index #9=w580, index #10=w579, index #11=w563, index #12=w562, index #13=w561, index #14=w539, index #15=w538) -> (element #1=w604:u16, element #2=w600:u16, element #3=w596:u16, element #4=w595:u16, element #5=w594:u16, element #6=w585:u16, element #7=w584:u16, element #8=w578:u16, element #9=w577:u16, element #10=w576:u16, element #11=w566:u16, element #12=w565:u16, element #13=w564:u16, element #14=w536:u16, element #15=w535:u16)
                  n119 = Select(t=myRIO_BRig_RT__Case_NonExp_stateList."SendData" ("Enum"), s=w549, f=w550) -> (s? t:f=w546:T1)
                  n120 = To Double Precision Float(number=w536) -> (double precision float=w534:dbl)
                  n121 = To Double Precision Float(number=w535) -> (double precision float=w533:dbl)
                  n122 = To Double Precision Float(number=w604) -> (double precision float=w603:dbl)
                  n123 = To Double Precision Float(number=w600) -> (double precision float=w602:dbl)
                  n124 = To Double Precision Float(number=w585) -> (double precision float=w587:dbl)
                  n125 = To Double Precision Float(number=w584) -> (double precision float=w586:dbl)
                  n126 = To Double Precision Float(number=w578) -> (double precision float=w575:dbl)
                  n127 = To Double Precision Float(number=w577) -> (double precision float=w574:dbl)
                  n128 = To Double Precision Float(number=w576) -> (double precision float=w573:dbl)
                  n129 = To Unsigned Word Integer(number=w537) -> (unsigned 16bit integer=w590:u16)
                  n130 = To Double Precision Float(number=w566) -> (double precision float=w567:dbl)
                  n131 = To Double Precision Float(number=w565) -> (double precision float=w568:dbl)
                  n132 = To Double Precision Float(number=w564) -> (double precision float=w569:dbl)
                  n133 = Not Equal To 0?(x=w594) -> (x != 0?=w591:bool)
                  n134 = Not Equal To 0?(x=w596) -> (x != 0?=w593:bool)
                  n135 = Not Equal To 0?(x=w595) -> (x != 0?=w592:bool)
                  n136 = Divide(x=w603, y=w601) -> (x/y=w530:dbl)
                  n137 = Divide(x=w602, y=w601) -> (x/y=w529:dbl)
                  n138 = local read "get_countPerMS"() -> (w545:bool)
                  n139 = Multiply(x=w537, y=w534) -> (x*y=w543:dbl)
                  n140 = Multiply(x=w537, y=w533) -> (x*y=w541:dbl)
                  n141 = call "BRig_RT__Case_Idle__calc_FPGA_CueLed.vi"("input_FPGA_ms2count"=w537, "input_Tpeak"=w587, "input_Freq"=w586) -> ("output_laser_Npeak"=w583:u32, "output_laser_Nvalley"=w582:u32)  [unwired: 11 in]
                  n142 = call "BRig_RT__Case_Idle__calc_FPGA_laser.vi"("input_FPGA_ms2count"=w537, "input_Tpeak"=w575, "input_Freq"=w574, "input_Tshutter"=w573) -> ("output_laser_Npeak"=w572:u32, "output_laser_Nvalley"=w571:u32, "output_laser_Nshutter"=w570:u32)  [unwired: 9 in]
                  n143 = call "BRig_RT__Case_Idle__calc_FPGA_laser.vi"("input_FPGA_ms2count"=w537, "input_Tpeak"=w567, "input_Freq"=w568, "input_Tshutter"=w569) -> ("output_laser_Npeak"=w560:u32, "output_laser_Nvalley"=w559:u32, "output_laser_Nshutter"=w558:u32)  [unwired: 9 in]
                  n144 = local write "L_Power_l1"(w530) -> ()
                  n145 = local write "L_Power_l2"(w529) -> ()
                  n146 = call "myRIO__convert__Voltage_to_FPGAvalue.vi"("input_voltage"=w530) -> ("output_PortA"=w527:u16)  [unwired: 9 in, 1 out]
                  n147 = call "myRIO__convert__Voltage_to_FPGAvalue.vi"("input_voltage"=w529) -> ("output_PortA"=w528:u16)  [unwired: 9 in, 1 out]
                  n148 = Round Toward +Infinity(x=w543) -> (ceil(x): smallest int >= x=w542:dbl)
                  n149 = Round Toward +Infinity(x=w541) -> (ceil(x): smallest int >= x=w540:dbl)
                  n150 = To Unsigned Long Integer(number=w542) -> (unsigned 32bit integer=w532:u32)
                  n151 = To Unsigned Long Integer(number=w540) -> (unsigned 32bit integer=w531:u32)
                  n152 = Select(t=myRIO_BRig_RT__Case_NonExp_stateList."Get_FPGA_count_per_ms" ("Enum"), s=w545, f=w546) -> (s? t:f=w544:T1)
                  n153 = xnode "Read/Write Control"("FPGA VI Reference In"=w609, "error in"=w608, "audioAmp_L"=w554, "audioFreq_L_kHz"=w553, "audioAmp_R"=w552, "audioFreq_R_kHz"=w551, "AnaOut_0"=w527, "AnaOut_1"=w528, "CueLed_Baseline"=w593, "L1Led_Baseline"=w592, "L2Led_Baseline"=w591, "k1__counter_per_ms"=w590, "CueLed_nPeak"=w583, "CueLed_nValley"=w582, "LC_nPeak_l1"=w572, "LC_nValley_l1"=w571, "LC_nShutter_l1"=w570, "LC_nPeak_l2"=w560, "LC_nValley_l2"=w559, "LC_nShutter_l2"=w558, "Solenoid_nTotal_L"=w532, "Solenoid_nTotal_R"=w531) -> ("error out"=w607:errorcluster)  [unwired: 1 out]
                  n154 = local write "error out"(w607) -> ()
                }
                frame "Idle_2" {
                  w615 = FALSE
                  n155 = call "BRig_RT_panel_cue_v0,90.vi"("input_setValues"=w615, "input_dataExp"=w624) -> ("output_dataExp"=w625:u16[])  [unwired: 9 in]
                  n156 = call "BRig_RT_panel_ExpStruct_v0,96.vi"("input_setValues"=w615, "input_dataExp"=w625) -> ("output_dataExp"=w618:u16[])  [unwired: 9 in]
                  n157 = local read "comm_TCP_connect"() -> (w614:bool)
                  n158 = call "BRig_RT_panel_Laser1_v0,90.vi"("input_setValues"=w615, "input_dataExp"=w618, "input_dataLC"=w623) -> ("output_dataExp"=w617:u16[], "output_dataLC"=w620:u16[])  [unwired: 7 in]
                  n159 = Select(t=myRIO_BRig_RT__Case_NonExp_stateList."commTCP_connect" ("Enum"), s=w614, f=myRIO_BRig_RT__Case_NonExp_stateList."Idle_6" ("Enum")) -> (s? t:f=w612:T1)
                  n160 = call "BRig_RT_panel_Laser2_v0,90.vi"("input_setValues"=w615, "input_dataExp"=w617, "input_dataLC"=w620) -> ("output_dataExp"=w616:u16[], "output_dataLC"=w619:u16[])  [unwired: 7 in]
                  n161 = local read "comm_WebDAV_connect"() -> (w613:bool)
                  n162 = Select(t=myRIO_BRig_RT__Case_NonExp_stateList."TestConnection" ("Enum"), s=w613, f=w612) -> (s? t:f=w610:T1)
                }
                frame "Idle_6" {
                  n163 = local read "lick_Rising(F)_or_Falling(T)"() -> (w627:bool)
                  n164 = call "BRig_RT__Case_Idle__State_UploadSettings_checkFile.vi"("input_dataName"="dataExp") -> ("output_Iexist"=w636:bool)  [unwired: 9 in, 1 out]
                  n165 = xnode "Read/Write Control"("FPGA VI Reference In"=w629, "error in"=w628, "Rising(F)_or_Falling(T)"=w627) -> ()  [unwired: 2 out]
                  n166 = Select(t=myRIO_BRig_RT__Case_NonExp_stateList."UploadSettings_pre" ("Enum"), s=w636, f=myRIO_BRig_RT__Case_NonExp_stateList."Idle") -> (s? t:f=w634:T1)
                }
                frame "Cue_pre" {
                  n167 = call "BRig_RT__Case_Idle__State_Cue_pre__v2.vi"("input_dataExp"=w638, "input_dataMTrig"=w642) -> ("output_dataMTrig"=w641:u16[], "output_state"=w640:T1)  [unwired: 8 in]
                }
                frame "Cue" {
                  n168 = call "BRig_RT__Case_Idle__State_Cue__v2.vi"("input_cLick_R_prev"=w645, "input_cLick_R"=w646, "input_state"=w651, "input_cLick_L_prev"=w647, "input_cLick_L"=w648, "input_dataMTrig"=w652) -> ("output_dataMTrig"=w650:u16[], "output_state"=w649:T1)  [unwired: 4 in]
                }
                frame "RewardCalibration_pre" {
                  n169 = call "BRig_RT__Case_Idle__State_RewardCalibration_pre__v2.vi"("input_dataMTrig"=w654) -> ("output_dataMTrig"=w653:u16[])  [unwired: 26 in]
                }
                frame "RewardCalibration" {
                  n170 = call "BRig_RT__Case_Idle__State_RewardCalibration.vi"("input_state"=w659, "input_dataMTrig"=w661) -> ("output_dataMtrig"=w660:u16[], "output_state"=w658:T1)  [unwired: 8 in]
                }
                frame "TestConnection" {
                  n171 = local read "Host Password"() -> (w667:string)
                  n172 = local read "Host UserName"() -> (w668:string)
                  n173 = call "BRig_RT_comm_webdav_connect.vi"("input_password"=w667, "input_username"=w668) -> ("output_Iconnected"=w666:bool, "output_hSession"=w665:T4)  [unwired: 6 in, 2 out]
                  n174 = local write "comm_WebDAV_connect"(FALSE ("comm_WebDAV_connect")) -> ()
                  n175 = local write "comm_WebDAV"(w666) -> ()
                }
                frame "SendData" {
                  n176 = And(x=w677, y=w676) -> (x .and. y?=w675:bool)
                  n177 = case shown="True" w675 {
                    tunnel: w676 -> [_ w694]
                    tunnel: w682 -> [_ w693]
                    tunnel: w681 -> [_ w692]
                    tunnel: w679 -> [_ w690]
                    tunnel: w678 -> [_ w689]
                    frame False {
                      n178 = One Button Dialog(message="Unable to send data:\n Missing one or more\n connections") -> ()  [unwired: 1 in, 1 out]
                    }
                    frame True {
                      n179 = local read "Data Set Prefix"() -> (w695:string)
                      n180 = call "BRig_RT_comm_webdav_upload_all__v3.vi"("input_I_connected_webdav"=w694, "input_fileName_prefix"=w695, "input_hSession"=w693, "input_error"=w692, "input_True"=TRUE) -> ("output_nFilenames"=w696:i32, "output_arrFilenames"=w697:string[], "output_uploaded"=w698:bool[], "output_strCmd"=w691:string)  [unwired: 5 in, 2 out]
                      n181 = call "BRig_RT_comm_tcp_write_RTwrite.vi"("input_error"=w689, "input_packet"=w691, "input_hTCP"=w690) -> ()  [unwired: 5 in, 4 out]
                      n182 = call "BRig_RT_comm_webdav_upload_all_warnUser.vi"("input_n"=w696, "input_arrFilenames"=w697, "input_arrUploaded"=w698) -> ()  [unwired: 9 in]
                    }
                  }
                  n183 = local write "I_sendData"(FALSE ("I_sendData")) -> ()
                }
                frame "Get_FPGA_count_per_ms" {
                  # "Used to automatically determine how many FPGA cycles in 1 ms"
                  n184 = case shown="True" w711 {
                    selector: w711 -> [w713 _]
                    tunnel: w709 -> [_ w726]
                    tunnel: [w717 w726] -> w708
                    tunnel: w707 -> [w716 w724]
                    tunnel: w706 -> [w715 w723]
                    tunnel: [w714 w721] -> w701
                    tunnel: [w713 w720] -> w705
                    frame False {
                      n185 = Get Date/Time In Seconds() -> (seconds since 1Jan1904=w718:timestamp)
                      n186 = To Double Precision Float(number=w718) -> (double precision float=w717:dbl)
                      n187 = xnode "Read/Write Control"("FPGA VI Reference In"=w716, "error in"=w715, "timeTrial_trig"=TRUE ("timeTrial")) -> ("error out"=w714:errorcluster)  [unwired: 1 out]
                      n188 = local write "get_countPerMS"(w713) -> ()
                    }
                    frame True {
                      w722 = 1.0
                      n189 = Get Date/Time In Seconds() -> (seconds since 1Jan1904=w727:timestamp)
                      n190 = To Double Precision Float(number=w727) -> (double precision float=w728:dbl)
                      n191 = Subtract(x=w728, y=w726) -> (x-y=w725:dbl)
                      n192 = Less Or Equal?(x=w722, y=w725) -> (x <= y?=w720:bool)
                      n193 = case shown="True" w720 {
                        tunnel: w724 -> [_ w741]
                        tunnel: w723 -> [w729 w740]
                        tunnel: w722 -> [_ w731]
                        tunnel: [w729 w730] -> w721
                        frame False {
                        }
                        frame True {
                          n194 = xnode "Read/Write Control"("FPGA VI Reference In"=w741, "error in"=w740) -> ("FPGA VI Reference Out"=w738:refnum<k20>, "error out"=w737:errorcluster, "timeTrial_count"=w732)
                          n195 = Multiply(x=w731, y=1000.0) -> (x*y=w735:dbl)
                          n196 = To Double Precision Float(number=w732) -> (double precision float=w734:dbl)
                          n197 = Divide(x=w734, y=w735) -> (x/y=w736:dbl)
                          n198 = local write "FPGA_count2ms"(w736) -> ()
                          n199 = xnode "Read/Write Control"("FPGA VI Reference In"=w738, "error in"=w737, "timeTrial_trig"=FALSE ("timeTrial")) -> ("error out"=w730:errorcluster)  [unwired: 1 out]
                        }
                      }
                    }
                  }
                  n200 = Select(t=myRIO_BRig_RT__Case_NonExp_stateList."Idle" ("Enum"), s=w705, f=w703) -> (s? t:f=w702:T1)
                  n201 = local write "error out"(w701) -> ()
                }
                frame "End" {
                }
                frame "commTCP_connect" {
                  n202 = local read "comm_TCP_connect"() -> (w751:bool)
                  n203 = case shown="True" w758 {
                    tunnel: w757 -> [w768 w777]
                    tunnel: [w767 w773] -> w755
                    tunnel: [w766 w770] -> w747
                    tunnel: [w765 w771] -> w756
                    tunnel: w754 -> [_ w778]
                    frame False {
                      n204 = call "BRig_RT_comm_tcp_connect_RTwrite.vi"("input_error"=w768) -> ("output_error"=w765:errorcluster, "output_connected"=w766:bool, "output_hTCP"=w767:refnum<k5>)  [unwired: 8 in]
                    }
                    frame True {
                      n205 = call "BRig_RT_comm_tcp_write_RTwrite.vi"("input_error"=w777, "input_packet"="<test>", "input_hTCP"=w778) -> ("output_error"=w772:errorcluster, "output_I_NotDisconnected"=w769:bool, "output_I_write"=w775:bool, "output_hTCP"=w774:refnum<k5>)  [unwired: 5 in]
                      n206 = case shown="False" w775 {
                        selector: w775 -> [_ w789]
                        tunnel: w774 -> [w784 w791]
                        tunnel: [w779 w791] -> w773
                        tunnel: w772 -> [w783 w790]
                        tunnel: [w781 w790] -> w771
                        tunnel: [w780 w789] -> w770
                        tunnel: w769 -> [w785 _]
                        frame False {
                          n207 = case shown="True" w785 {
                            tunnel: w784 -> [_ w788]
                            tunnel: w783 -> [w786 w787]
                            tunnel: [w786 w787] -> w782
                            frame False {
                            }
                            frame True {
                              n208 = TCP Close Connection(connection ID=w788, error in (no error)=w787) -> ()  [unwired: 1 in, 2 out]
                            }
                          }
                          n209 = call "BRig_RT_comm_tcp_connect_RTwrite.vi"("input_error"=w782) -> ("output_error"=w781:errorcluster, "output_connected"=w780:bool, "output_hTCP"=w779:refnum<k5>)  [unwired: 8 in]
                        }
                        frame True {
                        }
                      }
                    }
                  }
                  n210 = Not(x=w751) -> (.not. x?=w750:bool)
                  n211 = Or(x=w750, y=w747) -> (x .or. y?=w749:bool)
                  n212 = case shown="True" w749 {
                    tunnel: [w762 myRIO_BRig_RT__Case_NonExp_stateList."Idle" ("Enum")] -> w753
                    tunnel: w752 -> [w762 _]
                    frame False {
                    }
                    frame True {
                      n213 = local write "comm_TCP_connect"(FALSE) -> ()
                    }
                  }
                  n214 = local write "comm_TCP"(w747) -> ()
                }
              }
              n215 = case shown="True" w374 {
                tunnel: [w432 w433] -> w377
                tunnel: [w431 w434] -> w376
                tunnel: [w430 w435] -> w375
                tunnel: w373 -> [w432 _]
                tunnel: w372 -> [w431 _]
                tunnel: w371 -> [w430 _]
                tunnel: w370 -> [_ w435]
                tunnel: w369 -> [_ w434]
                tunnel: w368 -> [_ w433]
                frame False {
                }
                frame True {
                }
              }
              n216 = case shown="True" w364 {
                tunnel: [w426 w427] -> w363
                tunnel: [w425 w428] -> w362
                tunnel: [w424 w429] -> w361
                tunnel: w365 -> [w426 _]
                tunnel: w366 -> [w425 _]
                tunnel: w367 -> [w424 _]
                tunnel: w359 -> [_ w429]
                tunnel: w358 -> [_ w428]
                tunnel: w360 -> [_ w427]
                frame False {
                }
                frame True {
                }
              }
              n217 = flat-sequence {
                tunnel: w397 -> [w439]
                tunnel: w395 -> [w437]
                tunnel: [w439] -> w401
                tunnel: [w438] -> w400
                tunnel: [w437] -> w399
                tunnel: [w436] -> w398
                tunnel: w394 -> [w436]
                tunnel: [w451] -> w396
                tunnel: w401 -> [w451]
                tunnel: w400 -> [w450]
                tunnel: w399 -> [w448]
                tunnel: w398 -> [w443]
                tunnel: [w442] -> w393
                frame #0 {
                  n218 = Get Date/Time In Seconds() -> (seconds since 1Jan1904=w438:timestamp)
                }
                frame #1 {
                  # "threshold"
                  # "delta T [ms]"
                  # "delta T [s]"
                  n219 = To Double Precision Float(number=w450) -> (double precision float=w449:dbl)
                  n220 = To Double Precision Float(number=w448) -> (double precision float=w447:dbl)
                  n221 = Subtract(x=w449, y=w447) -> (x-y=w446:dbl)
                  n222 = Multiply(x=w446, y=1000.0) -> (x*y=w441:dbl)
                  n223 = Greater?(x=w441, y=5.0) -> (0:w440:bool)
                  n224 = local write "Threshold"(w440) -> ()
                  n225 = local write "tLoop"(w441) -> ()
                  n226 = Or(x=w440, y=w443) -> (x .or. y?=w442:bool)
                }
              }
              n227 = local read "START"() -> (w418:bool)
              n228 = local read "STOP_abort"() -> (w417:bool)
              n229 = local read "Laser1_LED"() -> (w355:bool)
              n230 = local read "Laser2_LED"() -> (w354:bool)
              n231 = call "BRig_RT_panel_manualTriggering_v0,90.vi"("input_dataMTrig"=w382) -> ("output_Solenoid_R"=w385:bool, "output_Solenoid_L"=w386:bool, "output_dataMTrig"=w392:u16[], "output_Audio_L"=w387:bool, "output_Audio_R"=w388:bool, "output_CueLed"=w389:bool, "output_Laser_l1"=w390:bool, "output_Laser_l2"=w391:bool)  [unwired: 11 in]
              n232 = Or(x=w418, y=w417) -> (x .or. y?=w416:bool)
              n233 = Select(t=myRIO_BRig_RT__Case_NonExp_stateList."End" ("Enum"), s=w416, f=w415) -> (s? t:f=w414:T1)
              n234 = xnode "Read/Write Control"("FPGA VI Reference In"=w409, "error in"=w408, "A1_SR"=w385, "A3_SL"=w386, "audioTrigger_L"=w387, "audioTrigger_R"=w388, "LC_Laser_l1"=w390, "LC_Laser_l2"=w391, "CueLed_Event"=w389, "L1Led_ON"=w355, "L2Led_ON"=w354) -> ("FPGA VI Reference Out"=w420:refnum<k20>, "error out"=w397:errorcluster)
              n235 = node-c288() -> ()  [unwired: 1 in, 1 out]
            }
            n236 = node-c288(w349) -> ()  [unwired: 1 out]
            n237 = flat-sequence {
              tunnel: w343 -> [w353]
              tunnel: [w353] -> w342
              tunnel: w341 -> [w352]
              tunnel: [w352] -> w340
              frame #0 {
                w351 = FALSE
                n238 = local write "STOP_endBlock"(w351) -> ()
                n239 = local write "STOP_endTrial"(w351) -> ()
              }
            }
          }
          frame True {
            w853 = ".csv" ("string")
            w883 = ""
            w892 = u8 0
            w893 = u16 0 ("AudioLeft_phase_inc")
            w894 = FALSE
            # "Clear local files"
            # "empty array"
            # "empty array"
            # "buffer_dataBlock"
            # "buffer_dataTrial"
            # "nColumns dataBlock"
            # "nColumns dataTrial"
            # "buffer_dataBlock"
            # "buffer_dataTrial"
            # "nColumns\ndataBlock"
            # "nColumns\ndataTrial"
            # "original dataExp and dataLC"
            # "dataLick"
            # "dataTrial"
            # "dataBlock"
            # "dataCurrent"
            # "arrTrig"
            # "time stamp"
            # "dummyState counter"
            # "dataTrial"
            # "dataLick"
            # "dataLC"
            # "dataLC"
            # "dataBlock"
            # "dataMTrig"
            # "dataMTrig"
            # "dataExp"
            # "dataExp"
            # "dataCurrent"
            # "state"
            n240 = flat-sequence {
              tunnel: [w990] -> w821
              tunnel: [w989] -> w826
              tunnel: [w998] -> w840
              tunnel: [w997] -> w839
              tunnel: [myRIO_BRig_RT__Case_Exp_stateList."Start1" ("Enum")] -> w838
              tunnel: [w995] -> w837
              tunnel: [u16 0] -> w836
              tunnel: [w993] -> w835
              tunnel: [w992] -> w834
              tunnel: [w991] -> w833
              tunnel: [w1000] -> w849
              tunnel: [w1001] -> w850
              tunnel: [w1002] -> w900
              tunnel: [w1003] -> w902
              tunnel: [w1004] -> w903
              tunnel: [w1005] -> w904
              tunnel: [w1006] -> w905
              tunnel: [w1007] -> w906
              tunnel: w840 -> [w1007]
              tunnel: w839 -> [w1006]
              tunnel: w838 -> [w1005]
              tunnel: w837 -> [w1004]
              tunnel: w836 -> [w1003]
              tunnel: w835 -> [w1002]
              tunnel: w834 -> [w1001]
              tunnel: w833 -> [w1000]
              tunnel: [w999] -> w831
              frame #0 {
                n241 = call "BRig_dataBlock_init.vi"() -> ("output_nCol"=w989:i32, "output_dataBlock"=w991:u16[][])  [unwired: 10 in]
                n242 = call "BRig_dataCurrent_init.vi"() -> ("output_dataCurrent"=w998:u16[])  [unwired: 11 in]
                n243 = call "BRig_dataLick_init.vi"() -> ("output_dataLick"=w997:u16[][])  [unwired: 11 in]
                n244 = call "BRig_dataTrial_init.vi"() -> ("output_nCol"=w990:i32, "output_dataTrial"=w992:u16[][])  [unwired: 10 in]
                n245 = Get Date/Time In Seconds() -> (seconds since 1Jan1904=w988:timestamp)
                n246 = To Double Precision Float(number=w988) -> (double precision float=w995:dbl)
                n247 = call "BRig_arrTrig_init.vi"() -> ("output_arrTrig"=w993:bool[])  [unwired: 11 in]
              }
              frame #1 {
                w999 = u32 2 ("milliseconds to wait")
                n248 = Wait (ms)(milliseconds to wait=w999) -> ()  [unwired: 1 out]
              }
            }
            n249 = call "BRig_comm_webdav_myrioFolder.vi"() -> ("output_myrioFolder"=w854:string)  [unwired: 11 in]
            n250 = flat-sequence {
              tunnel: w828 -> [w969]
              tunnel: [w969] -> w827
              tunnel: w827 -> [w978]
              tunnel: [w976] -> w809
              tunnel: [w975] -> w825
              tunnel: [w972] -> w824
              tunnel: w826 -> [w971]
              tunnel: w821 -> [w970]
              tunnel: [w978] -> w823
              tunnel: w823 -> [w980]
              tunnel: [w980] -> w822
              tunnel: w822 -> [w986]
              tunnel: w821 -> [w985]
              tunnel: [w983] -> w816
              tunnel: [w981] -> w819
              tunnel: [w986] -> w820
              tunnel: [w987] -> _
              tunnel: w820 -> [w987]
              frame #0 {
                n251 = Wait (ms)(milliseconds to wait=w969) -> ()  [unwired: 1 out]
              }
              frame #1 {
                w973 = u16 0 ("element")
                n252 = Initialize Array(w973, 8 ("dimension size")) -> (w976:u16[])
                n253 = Initialize Array(w973, 100 ("dimension size"), w970) -> (w975:u16[][])
                n254 = Initialize Array(w973, 10 ("dimension size"), w971) -> (w972:u16[][])
              }
              frame #2 {
                n255 = Wait (ms)(milliseconds to wait=w980) -> ()  [unwired: 1 out]
              }
              frame #3 {
                n256 = Increment(x=w985) -> (x+1=w982:i32)
                n257 = To Unsigned Long Integer(number=w982) -> (unsigned 32bit integer=w981:u32)
                n258 = Initialize Array(u16 0 ("element"), w982) -> (w983:u16[])
              }
              frame #4 {
                n259 = Wait (ms)(milliseconds to wait=w987) -> ()  [unwired: 1 out]
              }
            }
            n260 = local write "stop_TimedLoop"(FALSE ("stop_TimedLoop")) -> ()
            n261 = RT FIFO Create(0:"dataTrialOrBlock" ("name (unnamed)"), 1:w816, 4:u32 40 ("size (10)"), 6:w819, 7:T8 {"read mode"=enum."blocking", "write mode"=enum."blocking"} ("r/w modes (polling,polling)")) -> (8:w818:refnum<k33>, 11:w817:errorcluster)  [unwired: 3 in, 1 out]
            n262 = RT FIFO Create(0:"dataAnalog" ("name (unnamed)"), 1:u16 0 ("element"), 4:u32 1000 ("size (10)")) -> (8:w804:refnum<k33>, 11:w803:errorcluster)  [unwired: 5 in, 1 out]
            n263 = Concatenate Strings(w854, "dataTrial" ("input_filename"), w853) -> (w855:string)
            n264 = Concatenate Strings(w854, "dataBlock" ("input_filename"), w853) -> (w856:string)
            n265 = String To Path(string=w855) -> (path=w859:path)
            n266 = String To Path(string=w856) -> (path=w851:path)
            n267 = flat-sequence {
              tunnel: [w1008] -> w832
              tunnel: w831 -> [w1008]
              tunnel: w832 -> [w1009]
              tunnel: [w1009] -> w829
              tunnel: w846 -> [w1012]
              tunnel: w797 -> [w1011]
              tunnel: [w1010] -> w830
              tunnel: w829 -> [w1010]
              tunnel: [w1016] -> _
              tunnel: w845 -> [w1016]
              tunnel: w844 -> [w1015]
              tunnel: w843 -> [w1014]
              tunnel: [w1013] -> w828
              tunnel: w830 -> [w1013]
              frame #0 {
                n268 = call "BRig_RT__Case_Exp__clearLocalFolder.vi"() -> ()  [unwired: 12 in]
              }
              frame #1 {
                n269 = Wait (ms)(milliseconds to wait=w1009) -> ()  [unwired: 1 out]
              }
              frame #2 {
                n270 = call "BRig_RT__Case_Exp__State_start__sendExpData_saveData.vi"("input_dataLC"=w1012, "input_dataExp"=w1011) -> ()  [unwired: 10 in]
              }
              frame #3 {
                n271 = call "BRig_RT__Case_Exp__State_start__sendExpData_uploadData__v2.vi"("input_error"=w1016, "input_hSession"=w1015, "input_connected"=w1014) -> ()  [unwired: 8 in, 1 out]
              }
            }
            n272 = call "BRig_RT__Case_Exp__comm_tcp__data_other.vi"("input_strState"=w883, "input_strAccum"=w883, "input_error"=w888, "input_hTCP"=w889, "input_I_connected_TCP"=w890) -> ("output_strAccum"=w884:string, "output_error"=w885:errorcluster, "output_hTCP"=w886:refnum<k5>, "output_I_connect_TCP"=w887:bool)  [unwired: 3 in]
            n273 = node-c288() -> (w912:T5)  [unwired: 4 in]
            n274 = timed-loop {
              timing: w912 -> [_]
              timing-out: [_] -> w911
              shift-right: [w1210] -> _
              shift-left: w904 -> [w1165]
              tunnel: w899 -> [w1254]
              tunnel: w898 -> [w1234]
              shift-right: [w1198] -> _
              shift-left: w910 -> [w1253]
              shift-right: [w1197] -> _
              shift-left: w909 -> [w1252]
              tunnel: [w1245] -> w891
              tunnel: [w1246] -> w908
              shift-right: [w1208] -> w879
              shift-left: w906 -> [w1182]
              shift-right: [w1251] -> w880
              shift-left: w797 -> [w1184]
              shift-right: [w1228] -> w882
              shift-left: w896 -> [w1185]
              shift-right: [w1249] -> _
              shift-left: w849 -> [w1250]
              shift-right: [w1247] -> w881
              shift-left: w846 -> [w1248]
              shift-right: [w1204] -> w878
              shift-left: w905 -> [w1211]
              shift-right: [w1244] -> _
              shift-left: w850 -> [w1183]
              tunnel: w903 -> [w1243]
              shift-right: [w1217] -> _
              shift-left: u16 0 -> [w1216]
              shift-right: [w1237] -> _
              shift-left: w902 -> [w1238]
              shift-right: [w1235] -> _
              shift-left: w900 -> [w1236]
              shift-right: [w1229] -> _
              shift-left: FALSE -> [w1231]
              shift-right: [w1173] -> w870
              shift-left: w887 -> [w1192]
              shift-right: [w1172] -> w869
              shift-left: w886 -> [w1191]
              shift-right: [w1170] -> w868
              shift-left: w885 -> [w1190]
              shift-right: [w1171] -> _
              shift-left: w884 -> [w1189]
              shift-right: [w1179] -> w875
              shift-left: w845 -> [w1179]
              shift-right: [w1181] -> w873
              shift-left: w843 -> [w1181]
              shift-right: [w1180] -> w874
              shift-left: w844 -> [w1180]
              shift-right: [w1178] -> _
              shift-left: _ -> [w1176]
              shift-right: [w1177] -> _
              shift-left: _ -> [w1175]
              tunnel: [w1174] -> w862
              tunnel: w818 -> [w1168]
              tunnel: w817 -> [w1167]
              tunnel: w816 -> [w1166]
              tunnel: w804 -> [w1164]
              tunnel: w803 -> [w1163]
              tunnel: w797 -> [w1162]
              stop <- w1174 stop-if-true
              # "iOccurrence"
              # "index"
              # "resetOccurrence?\ndataAnalog"
              # "dataLick"
              # "dataLick"
              # "dummyState counter"
              # "dummyState counter"
              # "iOccurrence"
              # "arrTrig"
              # "arrTrig"
              # "CueLed"
              # "LC_Laser_l2"
              # "LC_Event_l2"
              # "LC_Laser_l1"
              # "LC_Event_l1"
              # "iState"
              # "dataAnalog"
              # "index"
              # "manual triggering"
              # "dataTrial"
              # "dataBlock"
              # "dataExp"
              # "dataCurrent"
              # "time stamp"
              # "audio__L\naudio__R"
              # "dataLC"
              # "solenoid__R"
              # "solenoid__L"
              # "Did a lick occur?"
              # "Update lick counter"
              # "state"
              # "state"
              n275 = node-c288() -> ()  [unwired: 1 in, 1 out]
              n276 = local write "cState"(w1165) -> ()
              n277 = flat-sequence {
                tunnel: w1234 -> [w1255]
                tunnel: [w1256] -> w1232
                tunnel: [w1255] -> w1233
                frame #0 {
                  n278 = Get Date/Time In Seconds() -> (seconds since 1Jan1904=w1256:timestamp)
                }
              }
              n279 = xnode "Read/Write Control"("FPGA VI Reference In"=w1254, "error in"=w1233) -> ("FPGA VI Reference Out"=w1240:refnum<k20>, "error out"=w1239:errorcluster, "A2_LickL"=w1198, "A4_LickR"=w1197)
              n280 = local write "A2"(w1198) -> ()
              n281 = local write "A4"(w1197) -> ()
              n282 = Greater?(x=w1198, y=w1253) -> (0:w1206:bool)
              n283 = Greater?(x=w1197, y=w1252) -> (0:w1205:bool)
              n284 = Or(x=w1206, y=w1205) -> (x .or. y?=w1207:bool)
              n285 = case shown="\"initTrial2\"" w1165 {
                selector: w1165 -> [_ _ _ _ _ _ _ _ _ _ _ _ _ w1456 _ w1485 _ w1517 _ w1543 _ w1587 _ w1627 _ w1647 _ w1685 _ w1727 _ _ _ _ w1846 _ w1870 w1901 w1922 w1947 _ w2004 w2014 _]
                tunnel: [myRIO_BRig_RT__Case_Exp_stateList."Start2" ("Enum") myRIO_BRig_RT__Case_Exp_stateList."Start3" ("Enum") myRIO_BRig_RT__Case_Exp_stateList."saveSettings1" ("Enum") myRIO_BRig_RT__Case_Exp_stateList."initBlock" ("Enum") myRIO_BRig_RT__Case_Exp_stateList."initTrial_LC_ENL1" ("Enum") myRIO_BRig_RT__Case_Exp_stateList."initTrial" ("Enum") myRIO_BRig_RT__Case_Exp_stateList."initTrial2" ("Enum") myRIO_BRig_RT__Case_Exp_stateList."setSettings_Laser" ("Enum") myRIO_BRig_RT__Case_Exp_stateList."ENL1_pre" ("Enum") myRIO_BRig_RT__Case_Exp_stateList."initTrial_LC_Cue1" ("Enum") myRIO_BRig_RT__Case_Exp_stateList."initTrial_LC_Sel" ("Enum") myRIO_BRig_RT__Case_Exp_stateList."initTrial4" ("Enum") w1446 w1454 myRIO_BRig_RT__Case_Exp_stateList."ENL1Penalty" ("Enum") w1483 w1497 w1516 myRIO_BRig_RT__Case_Exp_stateList."Cue1Penalty" ("Enum") w1544 w1560 w1582 myRIO_BRig_RT__Case_Exp_stateList."SelectReward" ("Enum") w1626 myRIO_BRig_RT__Case_Exp_stateList."SelectRewardPost" ("Enum") w1646 myRIO_BRig_RT__Case_Exp_stateList."SelectWrong" ("Enum") w1684 myRIO_BRig_RT__Case_Exp_stateList."SelectTimeout" ("Enum") w1726 myRIO_BRig_RT__Case_Exp_stateList."saveData_dataTrial" ("Enum") w1761 w1796 w1835 w1846 myRIO_BRig_RT__Case_Exp_stateList."initBlock" ("Enum") w1868 w1902 w1921 w1946 myRIO_BRig_RT__Case_Exp_stateList."FreeReward" ("Enum") w2002 w2012 myRIO_BRig_RT__Case_Exp_stateList."FreeRewardPost" ("Enum")] -> w1210
                tunnel: w1207 -> [_ _ _ _ _ _ _ _ _ _ _ _ w1447 w1455 _ _ w1498 w1518 _ _ _ _ _ _ _ _ _ _ _ _ _ _ _ _ _ _ _ _ _ _ _ _ _ _]
                tunnel: w1206 -> [_ _ _ _ _ _ _ _ _ _ _ _ _ _ _ _ _ _ _ _ w1552 w1583 _ _ _ _ _ _ _ _ _ _ _ _ _ _ _ _ _ _ _ _ _ _]
                tunnel: w1205 -> [_ _ _ _ _ _ _ _ _ _ _ _ _ _ _ _ _ _ _ _ w1551 w1584 _ _ _ _ _ _ _ _ _ _ _ _ _ _ _ _ _ _ _ _ _ _]
                tunnel: w1182 -> [w1266 w1272 w1287 w1291 w1312 w1349 w1352 w1369 w1394 w1409 w1419 w1436 w1444 w1463 w1474 w1482 w1499 w1519 w1536 w1542 w1563 w1580 w1612 w1623 w1635 w1645 w1669 w1683 w1707 w1725 w1740 w1767 w1805 w1825 w1845 w1852 w1871 w1904 w1920 w1937 w1976 w2000 w2011 w2022]
                tunnel: w1184 -> [w1257 w1271 w1277 w1289 w1300 w1348 w1362 w1370 w1405 w1408 w1418 w1428 w1451 w1466 w1473 w1490 w1496 w1522 w1529 w1550 w1559 w1579 w1614 w1625 w1633 w1652 w1665 w1690 w1702 w1732 w1750 w1759 w1803 w1810 w1844 w1849 w1873 w1906 w1932 w1952 w1957 w2005 w2015 w2021]
                tunnel: [w1266 w1272 w1287 w1291 w1312 w1347 w1351 w1372 w1394 w1412 w1426 w1435 w1448 w1462 w1475 w1481 w1493 w1502 w1535 w1541 w1558 w1581 w1605 w1628 w1634 w1643 w1662 w1681 w1700 w1724 w1742 w1767 w1805 w1825 w1845 w1852 w1871 w1904 w1920 w1937 w1982 w2001 w2010 w2020] -> w1209
                tunnel: [w1257 w1271 w1276 w1289 w1300 w1348 w1362 w1370 w1405 w1408 w1418 w1428 w1451 w1466 w1473 w1490 w1496 w1522 w1529 w1550 w1559 w1579 w1614 w1625 w1633 w1652 w1665 w1690 w1702 w1732 w1750 w1756 w1803 w1809 w1844 w1849 w1873 w1906 w1932 w1952 w1958 w2005 w2015 w2021] -> w1251
                tunnel: [_ _ _ _ _ _ _ _ _ _ _ _ _ _ _ _ _ _ _ _ _ _ _ w1617 _ _ _ _ _ _ _ _ _ _ _ _ _ _ _ _ _ w1994 _ _] -> w1194
                tunnel: [_ _ _ _ _ _ _ _ _ _ _ _ _ _ _ _ _ _ _ _ _ _ _ w1616 _ _ _ _ _ _ _ _ _ _ _ _ _ _ _ _ _ w1995 _ _] -> w1193
                tunnel: w1250 -> [w1265 w1269 w1285 w1293 w1325 w1344 w1356 w1384 w1406 w1414 w1425 w1433 w1450 w1465 w1470 w1488 w1501 w1521 w1534 w1547 w1569 w1591 w1611 w1630 w1639 w1650 w1667 w1688 w1706 w1731 w1736 w1768 w1794 w1827 w1842 w1851 w1853 w1907 w1930 w1950 w1985 w2007 w2017 w2029]
                tunnel: [w1265 w1269 w1285 w1293 w1325 w1343 w1355 w1384 w1406 w1414 w1425 w1433 w1450 w1465 w1470 w1488 w1501 w1521 w1534 w1547 w1569 w1591 w1610 w1630 w1639 w1650 w1666 w1688 w1704 w1731 w1736 w1768 w1794 w1827 w1842 w1851 w1853 w1907 w1930 w1950 w1985 w2007 w2017 w2029] -> w1249
                tunnel: w1248 -> [w1258 w1270 w1286 w1292 w1320 w1350 w1366 w1385 w1407 w1413 w1420 w1434 w1449 w1464 w1471 w1489 w1500 w1520 w1533 w1549 w1568 w1592 w1613 w1629 w1642 w1651 w1671 w1689 w1713 w1730 w1749 w1758 w1806 w1829 w1843 w1848 w1872 w1905 w1931 w1951 w1986 w2008 w2018 w2030]
                tunnel: [w1258 w1270 w1286 w1292 w1320 w1350 w1366 w1385 w1407 w1413 w1420 w1434 w1449 w1464 w1471 w1489 w1500 w1520 w1533 w1549 w1568 w1592 w1613 w1629 w1642 w1651 w1671 w1689 w1713 w1730 w1749 w1757 w1806 w1829 w1843 w1848 w1872 w1905 w1931 w1951 w1986 w2008 w2018 w2030] -> w1247
                tunnel: [_ _ _ _ _ _ _ _ _ _ _ _ _ _ _ _ _ _ _ _ _ _ _ _ _ _ _ _ _ _ _ _ _ _ TRUE _ _ _ _ _ _ _ _ _] -> w1212
                tunnel: [_ _ _ _ _ _ _ _ _ _ _ _ _ _ _ _ _ w1504 _ _ _ _ _ _ _ _ _ _ _ _ _ _ _ _ _ _ _ _ _ _ _ _ _ _] -> w1242
                tunnel: [_ _ _ _ _ _ _ _ _ _ _ _ _ _ _ _ _ w1503 _ _ _ _ _ _ _ _ _ _ _ _ _ _ _ _ _ _ _ _ _ _ _ _ _ _] -> w1241
                tunnel: w1183 -> [w1263 w1268 w1283 w1290 w1324 w1342 w1361 w1386 w1398 w1415 w1424 w1432 w1443 w1453 w1467 w1487 w1495 w1507 w1531 w1546 w1567 w1571 w1602 w1624 w1640 w1649 w1664 w1687 w1705 w1729 w1748 w1766 w1804 w1826 w1840 w1850 w1857 w1884 w1929 w1949 w1980 w2006 w2016 w2028]
                tunnel: [w1263 w1268 w1283 w1290 w1324 w1341 w1354 w1371 w1392 w1411 w1423 w1431 w1442 w1452 w1467 w1487 w1494 w1506 w1531 w1546 w1567 w1570 w1601 w1624 w1640 w1649 w1661 w1687 w1699 w1729 w1747 w1766 w1804 w1826 w1840 w1850 w1857 w1884 w1929 w1949 w1980 w2006 w2016 w2028] -> w1244
                tunnel: w1243 -> [_ _ _ _ _ _ _ _ _ _ _ _ _ _ _ _ _ _ _ _ _ _ _ _ _ _ _ _ _ _ w1741 _ _ _ _ _ _ _ _ _ _ _ _ _]
                tunnel: w1240 -> [w1262 _ _ _ w1321 w1336 w1365 w1390 w1403 _ _ w1439 _ _ _ _ _ w1508 _ _ w1565 w1590 w1600 _ _ _ _ _ w1711 _ w1744 _ _ _ w1838 _ _ _ _ _ w1964 _ _ _]
                tunnel: w1239 -> [w1261 _ _ _ w1322 w1335 w1353 w1389 w1402 _ _ w1438 _ _ _ _ _ w1509 _ _ w1566 w1589 w1599 _ _ _ _ _ w1710 _ w1743 _ _ _ w1837 _ _ _ _ _ w1963 _ _ _]
                tunnel: [_ _ _ _ _ _ _ _ _ _ _ _ _ w1461 _ _ _ w1514 _ _ w1557 w1577 _ _ _ _ _ _ _ _ _ _ _ _ _ _ _ _ _ _ _ _ _ _] -> w1218
                tunnel: [_ _ _ _ _ _ _ _ _ _ _ _ _ w1460 _ _ _ w1513 _ _ w1556 w1576 _ _ _ _ _ _ _ _ _ _ _ _ _ _ _ _ _ _ _ _ _ _] -> w1199
                tunnel: [_ _ _ _ _ _ _ _ TRUE ("Recording") _ _ _ _ _ _ _ _ _ _ _ _ _ _ _ _ _ _ _ _ _ _ _ _ _ _ _ _ _ _ _ _ _ _ _] -> w1215
                tunnel: w1238 -> [_ _ _ _ _ _ _ _ _ _ _ _ _ _ _ _ _ _ _ _ _ _ _ _ _ _ _ _ _ _ _ _ _ _ _ _ w1869 w1900 w1927 w1934 _ _ _ _]
                tunnel: [_ _ _ _ _ _ _ _ _ _ _ _ _ _ _ _ _ _ _ _ _ _ _ _ _ _ _ _ _ _ _ _ _ _ _ _ w1867 w1899 w1925 w1935 _ _ _ _] -> w1237
                tunnel: w1236 -> [_ _ _ _ w1294 _ _ _ w1399 w1416 w1422 w1430 w1445 w1457 w1468 w1486 w1492 w1515 w1530 w1545 w1553 w1578 _ _ _ _ _ _ _ _ _ _ _ _ _ _ _ _ _ _ _ _ _ _]
                tunnel: [_ _ _ _ w1294 _ _ w1373 w1399 w1410 w1421 w1429 w1445 w1457 w1468 w1486 w1491 w1515 w1530 w1545 w1553 w1578 _ _ _ _ _ _ _ _ _ _ _ _ _ _ _ _ _ _ _ _ _ _] -> w1235
                tunnel: [_ _ _ _ _ _ _ _ _ _ _ _ _ w1459 _ _ _ w1512 _ _ w1555 w1575 _ _ _ _ _ _ _ _ _ _ _ _ _ _ _ _ _ _ _ _ _ _] -> w1222
                tunnel: [_ _ _ _ _ _ _ _ _ _ _ _ _ w1458 _ _ _ w1511 _ _ w1554 w1574 _ _ _ _ _ _ _ _ _ _ _ _ _ _ _ _ _ _ _ _ _ _] -> w1223
                tunnel: [_ _ _ _ _ _ _ _ _ _ _ _ _ _ _ _ _ w1505 _ _ _ _ _ _ _ _ _ _ _ _ _ _ _ _ _ _ _ _ _ _ _ _ _ _] -> w1225
                tunnel: [_ _ "<S,S>" ("string") _ _ _ _ _ w1393 _ _ _ _ _ _ _ _ _ _ _ _ _ w1603 _ _ _ w1660 _ w1698 _ w1739 _ _ w1821 _ _ _ _ _ _ _ _ _ _] -> w1188
                tunnel: w1185 -> [_ _ _ _ _ _ _ _ _ _ _ _ _ _ _ _ _ _ _ _ _ _ _ _ _ _ _ _ _ _ _ _ _ _ _ _ _ _ _ _ w1971 _ _ _]
                tunnel: w1181 -> [_ _ _ _ _ _ _ _ _ _ _ _ _ _ _ _ _ _ _ _ _ _ _ _ _ _ _ _ _ _ _ _ _ w1820 _ _ _ _ _ _ _ _ _ _]
                tunnel: w1180 -> [_ _ _ _ _ _ _ _ _ _ _ _ _ _ _ _ _ _ _ _ _ _ _ _ _ _ _ _ _ _ _ _ _ _ _ _ _ _ _ _ _ _ _ _]
                tunnel: w1179 -> [_ _ _ _ _ _ _ _ _ _ _ _ _ _ _ _ _ _ _ _ _ _ _ _ _ _ _ _ _ _ _ _ _ _ _ _ _ _ _ _ _ _ _ _]
                tunnel: [_ _ _ _ _ _ _ _ _ _ _ _ _ _ _ _ _ _ _ _ _ _ _ _ _ _ _ _ _ _ _ w1760 _ _ _ _ _ _ _ _ _ _ _ _] -> w1178
                tunnel: [_ _ _ _ _ _ _ _ _ _ _ _ _ _ _ _ _ _ _ _ _ _ _ _ _ _ _ _ _ _ _ w1765 _ _ _ _ _ _ _ _ _ _ _ _] -> w1177
                tunnel: w1176 -> [_ _ _ _ _ _ _ _ _ _ _ _ _ _ _ _ _ _ _ _ _ _ _ _ _ _ _ _ _ _ _ w1764 _ _ _ _ _ _ _ _ _ _ _ _]
                tunnel: w1175 -> [_ _ _ _ _ _ _ _ _ _ _ _ _ _ _ _ _ _ _ _ _ _ _ _ _ _ _ _ _ _ _ w1755 _ _ _ _ _ _ _ _ _ _ _ _]
                tunnel: w1168 -> [_ _ _ _ _ _ _ _ _ _ _ _ _ _ _ _ _ _ _ _ _ _ _ _ _ _ _ _ _ _ _ _ _ _ _ _ w1864 w1887 _ _ _ _ _ _]
                tunnel: w1167 -> [_ _ _ _ _ _ _ _ _ _ _ _ _ _ _ _ _ _ _ _ _ _ _ _ _ _ _ _ _ _ _ _ _ _ _ _ w1863 w1886 _ _ _ _ _ _]
                tunnel: w1166 -> [_ _ _ _ _ _ _ _ _ _ _ _ _ _ _ _ _ _ _ _ _ _ _ _ _ _ _ _ _ _ _ _ _ _ _ _ w1861 w1885 _ _ _ _ _ _]
                tunnel: w1162 -> [_ _ _ _ _ _ _ _ _ _ _ _ _ _ _ _ _ _ _ _ _ _ _ _ _ _ _ _ _ _ _ _ _ w1815 _ _ _ _ _ _ _ _ _ _]
                frame "Start1", Default {
                  w1260 = FALSE ("SelectionState")
                  n286 = xnode "Read/Write Control"("FPGA VI Reference In"=w1262, "error in"=w1261, "SelectionState"=w1260, "LR_reward_Laser_l1"=w1260, "LR_wrong_Laser_l1"=w1260, "LR_reward_Event_l1"=w1260, "LR_wrong_Event_l1"=w1260, "Left(F)_or_Right(T)"=w1260, "SelectionState"=w1260, "LR_reward_Laser_l2"=w1260, "LR_wrong_laser_l2"=w1260, "LR_reward_Event_l2"=w1260, "LR_wrong_Event_l2"=w1260, "LC_Event_l1"=w1260, "LC_Laser_l1"=w1260, "LC_Laser_l2"=w1260, "LC_Event_l2"=w1260, "CueLed_Event"=w1260) -> ("error out"=w1259:errorcluster)  [unwired: 1 out]
                  n287 = local write "error out"(w1259) -> ()
                }
                frame "Start2" {
                }
                frame "Start3" {
                  w1273 = u16 0 ("new element/subarray")
                  w1278 = 0.0 ("BTPR_avg_L")
                  w1281 = FALSE ("SolenoidReward")
                  w1279 = u16 0 ("BTPR_block")
                  w1282 = u16 0 ("nRewards_cur")
                  # "Goal:\nPrepare dataCurrent"
                  n288 = call "BRig_dataExp_FreeReward_c_L.vi"() -> ("output_FreeReward_c_L"=w1275:i32)  [unwired: 11 in]
                  n289 = call "BRig_dataExp_FreeReward_c_R.vi"() -> ("output_FreeReward_c_R"=w1274:i32)  [unwired: 11 in]
                  n290 = local write "nRewards_cur"(w1282) -> ()
                  n291 = local write "nRewards_total"(w1282) -> ()
                  n292 = local write "nRewards_Left"(w1282) -> ()
                  n293 = local write "nRewards_Right"(w1282) -> ()
                  n294 = local write "BUR_target"(w1282) -> ()
                  n295 = local write "TpB_target"(w1282) -> ()
                  n296 = local write "iBlock"(w1282) -> ()
                  n297 = local write "iTrial"(w1282) -> ()
                  n298 = local write "nTrial"(w1282) -> ()
                  n299 = local write "SolenoidReward"(w1281) -> ()
                  n300 = local write "allReward_L"(w1281) -> ()
                  n301 = local write "allReward_R"(w1281) -> ()
                  n302 = Replace Array Subset(array=w1277, new element #1=w1273, index #1=w1275, new element #2=w1273, index #2=w1274) -> (w1276:u16[])
                  n303 = local write "FreeReward_c_L"(w1273) -> ()
                  n304 = local write "FreeReward_c_R"(w1273) -> ()
                  n305 = local write "BTPR_block"(w1279) -> ()
                  n306 = local write "T2R_block"(w1279) -> ()
                  n307 = local write "BTPR_avg_L"(w1278) -> ()
                  n308 = local write "BTPR_avg_R"(w1278) -> ()
                  n309 = local write "T2R_avg_L"(w1278) -> ()
                  n310 = local write "T2R_avg_R"(w1278) -> ()
                }
                frame "saveSettings1" {
                }
                frame "setSettings_Laser" {
                  n311 = call "BRig_dataExp_LED_baseline_Cue.vi"() -> ("output_LED_baseline_Cue"=w1309:i32)  [unwired: 11 in]
                  n312 = call "BRig_dataExp_LED_baseline_l1.vi"() -> ("output_LED_baseline_l1"=w1310:i32)  [unwired: 11 in]
                  n313 = call "BRig_dataExp_LED_baseline_l2.vi"() -> ("output_LED_baseline_l2"=w1308:i32)  [unwired: 11 in]
                  n314 = call "BRig_dataExp_I_anySelect.vi"() -> ("output_I_anySelect"=w1302:i32)  [unwired: 11 in]
                  n315 = call "BRig_dataExp_I_trialUntilReward.vi"() -> ("output_I_trialUntilReward"=w1301:i32)  [unwired: 11 in]
                  n316 = local read "FPGA_count2ms"() -> (w1319:dbl)
                  n317 = call "BRig_RT__Case_Exp__State_setLaserSettings.vi"("input_FPGA_count2ms"=w1319, "input_dataExp"=w1300, "input_dataLC"=w1320) -> ("output_LR_nTotal_l1"=w1318:u32, "output_LR_nTotal_l2"=w1317:u32, "output_LR_reward_nDelay_l1"=w1316:u32, "output_LR_wrong_nDelay_l1"=w1315:u32, "output_LR_reward_nDelay_l2"=w1314:u32, "output_LR_wrong_nDelay_l2"=w1313:u32)  [unwired: 11 in]
                  n318 = Index Array(array=w1300, index #1=w1309, index #2=w1310, index #3=w1308, index #4=w1302, index #5=w1301) -> (element #1=w1307:u16, element #2=w1306:u16, element #3=w1305:u16, element #4=w1304:u16, element #5=w1303:u16)
                  n319 = Not Equal To 0?(x=w1306) -> (x != 0?=w1298:bool)
                  n320 = Not Equal To 0?(x=w1304) -> (x != 0?=w1296:bool)
                  n321 = Not Equal To 0?(x=w1307) -> (x != 0?=w1299:bool)
                  n322 = Not Equal To 0?(x=w1305) -> (x != 0?=w1297:bool)
                  n323 = Not Equal To 0?(x=w1303) -> (x != 0?=w1295:bool)
                  n324 = xnode "Read/Write Control"("FPGA VI Reference In"=w1321, "error in"=w1322, "LR_reward_nTotal_l1"=w1318, "LR_wrong_nTotal_l1"=w1318, "LR_reward_nTotal_l2"=w1317, "LR_wrong_nTotal_l2"=w1317, "LR_reward_nDelay_l1"=w1316, "LR_wrong_nDelay_l1"=w1315, "LR_reward_nDelay_l2"=w1314, "LR_wrong_nDelay_l2"=w1313, "CueLed_Baseline"=w1299, "L1Led_Baseline"=w1298, "L2Led_Baseline"=w1297, "I_allReward"=w1296, "ignoreWrong"=w1295) -> ("error out"=→"error out":errorcluster)  [unwired: 1 out]
                }
                frame "initBlock" {
                  w1326 = u16 0 ("BTPR_block")
                  n325 = local write "nRewards_cur"(u16 0 ("nRewards_cur")) -> ()
                  n326 = local write "BTPR_block"(w1326) -> ()
                  n327 = local write "T2R_block"(w1326) -> ()
                  n328 = call "BRig_RT__Case_Exp__State_initBlock.vi"("input_dataCurrent"=w1349, "input_dataExp"=w1348, "input_dataBlock"=w1344, "input_dataTrial"=w1342) -> ("output_iSpout"=w1333:u16, "output_speaker_amp_R"=w1337:u16, "output_iBlock"=w1332:u16, "output_speaker_freq_R"=w1338:u8, "output_BUR_target"=w1331:u16, "output_speaker_amp_L"=w1339:u16, "output_TpB_target"=w1346:u16, "output_speaker_freq_L"=w1340:u8, "output_dataCurrent"=w1347:u16[], "output_dataBlock"=w1343:u16[][], "output_dataTrial"=w1341:u16[][])  [unwired: 5 in]
                  n329 = Type Cast(type=enum16{"Left", "Right"}."Left", x=w1333) -> (*(type *) &x=w1328:enum16{"Left", "Right"})
                  n330 = Not Equal To 0?(x=w1333) -> (x != 0?=w1327:bool)
                  n331 = local write "cSpout"(w1328) -> ()
                  n332 = local write "iBlock"(w1332) -> ()
                  n333 = local write "BUR_target"(w1331) -> ()
                  n334 = local write "TpB_target"(w1346) -> ()
                  n335 = xnode "Read/Write Control"("FPGA VI Reference In"=w1336, "error in"=w1335, "Left(F)_or_Right(T)"=w1327, "audioFreq_L_kHz"=w1340, "audioAmp_L"=w1339, "audioFreq_R_kHz"=w1338, "audioAmp_R"=w1337) -> ("error out"=w1334:errorcluster)  [unwired: 1 out]
                  n336 = local write "error out"(w1334) -> ()
                }
                frame "initTrial" {
                  n337 = xnode "Read/Write Control"("FPGA VI Reference In"=w1365, "error in"=w1353, "SelectionState"=FALSE) -> ("error out"=w1364:errorcluster)  [unwired: 1 out]
                  n338 = call "BRig_RT__Case_Exp__State_initTrial__v2.vi"("input_dataCurrent"=w1352, "input_dataBlock"=w1356, "input_dataTrial"=w1361, "input_dataExp"=w1362) -> ("output_iTrial"=w1359:u16, "output_nTrial"=w1357:u16, "output_SolenoidReward"=w1360:bool, "output_dataCurrent"=w1351:u16[], "output_dataBlock"=w1355:u16[][], "output_dataTrial"=w1354:u16[][])  [unwired: 6 in]
                  n339 = local write "iTrial"(w1359) -> ()
                  n340 = local write "nTrial"(w1357) -> ()
                  n341 = local write "SolenoidReward"(w1360) -> ()
                  n342 = local write "error out"(w1364) -> ()
                }
                frame "initTrial2" {
                  n343 = call "BRig_RT__Case_Exp__State_initTrial2.vi"("input_dataCurrent"=w1369, "input_dataTrial"=w1386, "input_dataExp"=w1370, "input_dataBlock"=w1384, "input_dataLC"=w1385) -> ("output_L_Wrong_Laser_l2"=w1376:bool, "output_L_Wrong_Event_l2"=w1377:bool, "output_L_Power_l1"=w1375:dbl, "output_L_Reward_Laser_l2"=w1378:bool, "output_L_Power_l2"=w1374:dbl, "output_L_Reward_Event_l2"=w1379:bool, "output_dataCurrent"=w1372:u16[], "output_dataTrial"=w1371:u16[][], "output_L_Reward_Event_l1"=w1383:bool, "output_L_Reward_Laser_l1"=w1382:bool, "output_L_Wrong_Event_l1"=w1381:bool, "output_L_Wrong_Laser_l1"=w1380:bool)  [unwired: 3 in]
                  n344 = local write "L_Power_l1"(w1375) -> ()
                  n345 = call "myRIO__convert__Voltage_to_FPGAvalue.vi"("input_voltage"=w1375) -> ("output_PortA"=w1367:u16)  [unwired: 9 in, 1 out]
                  n346 = local write "L_Power_l2"(w1374) -> ()
                  n347 = call "myRIO__convert__Voltage_to_FPGAvalue.vi"("input_voltage"=w1374) -> ("output_PortA"=w1368:u16)  [unwired: 9 in, 1 out]
                  n348 = xnode "Read/Write Control"("FPGA VI Reference In"=w1390, "error in"=w1389, "AnaOut_0"=w1367, "AnaOut_1"=w1368, "LR_reward_Event_l1"=w1383, "LR_reward_Laser_l1"=w1382, "LR_wrong_Event_l1"=w1381, "LR_wrong_Laser_l1"=w1380, "LR_reward_Event_l2"=w1379, "LR_reward_Laser_l2"=w1378, "LR_wrong_Event_l2"=w1377, "LR_wrong_laser_l2"=w1376) -> ("error out"=w1387:errorcluster)  [unwired: 1 out]
                  n349 = local write "error out"(w1387) -> ()
                  n350 = call "BRig_arrTrig_init.vi"() -> ("output_arrTrig"=w1373:bool[])  [unwired: 11 in]
                }
                frame "initTrial4" {
                  # "resetOccurrence?\ndataAnalog"
                  n351 = local read "FPGA_count2ms"() -> (w1395:dbl)
                  n352 = local read "lick_Rising(F)_or_Falling(T)"() -> (w1391:bool)
                  n353 = local read "Recording"() -> (w1397:bool)
                  n354 = call "BRig_RT_comm_tcp_write_RTwrite__RunState_Trial_start.vi"("input_dataCurrent"=w1394) -> ("output_strCmd"=w1393:string)  [unwired: 10 in]
                  n355 = call "BRig_RT__Case_Exp__State_initTrial4.vi"("input_Recording"=w1397, "input_FPGA_count2ms"=w1395, "input_dataTrial"=w1398) -> ("output_Solenoid_nTotal"=w1396:u32, "output_dataTrial"=w1392:u16[][])  [unwired: 7 in]
                  n356 = xnode "Read/Write Control"("FPGA VI Reference In"=w1403, "error in"=w1402, "Solenoid_nTotal_L"=w1396, "Solenoid_nTotal_R"=w1396, "A6_Act"=w1397, "Rising(F)_or_Falling(T)"=w1391) -> ("error out"=w1401:errorcluster)  [unwired: 1 out]
                  n357 = local write "error out"(w1401) -> ()
                }
                frame "initTrial_LC_ENL1" {
                  n358 = call "BRig_RT__Case_Exp__State_initTrial__LC_ENL.vi"("input_arrTrig"=w1416, "input_dataTrial"=w1415, "input_dataExp"=w1408, "input_dataLC"=w1413, "input_dataCurrent"=w1409) -> ("output_dataTrial"=w1411:u16[][], "output_dataCurrent"=w1412:u16[], "output_arrTrig"=w1410:bool[])  [unwired: 4 in]
                }
                frame "initTrial_LC_Cue1" {
                  n359 = call "BRig_RT__Case_Exp__State_initTrial__LC_Cue.vi"("input_arrTrig"=w1422, "input_dataTrial"=w1424, "input_dataExp"=w1418, "input_dataLC"=w1420, "input_dataCurrent"=w1419) -> ("output_dataTrial"=w1423:u16[][], "output_dataCurrent"=w1426:u16[], "output_arrTrig"=w1421:bool[])  [unwired: 4 in]
                }
                frame "initTrial_LC_Sel" {
                  n360 = call "BRig_RT__Case_Exp__State_initTrial__LC_Select.vi"("input_arrTrig"=w1430, "input_dataTrial"=w1432, "input_dataExp"=w1428, "input_dataLC"=w1434, "input_dataCurrent"=w1436) -> ("output_dataTrial"=w1431:u16[][], "output_dataCurrent"=w1435:u16[], "output_arrTrig"=w1429:bool[])  [unwired: 4 in]
                  n361 = xnode "Read/Write Control"("FPGA VI Reference In"=w1439, "error in"=w1438, "A6_Act"=FALSE) -> ("error out"=w1440:errorcluster)  [unwired: 1 out]
                  n362 = local write "error out"(w1440) -> ()
                }
                frame "ENL1_pre" {
                  n363 = call "BRig_RT__Case_Exp__State_ENLPre.vi"("input_I_lick"=w1447, "input_dataTrial"=w1443, "input_dataCurrent"=w1444) -> ("output_dataTrial"=w1442:u16[][], "output_dataCurrent"=w1448:u16[], "output_state"=w1446:T2)  [unwired: 6 in]
                }
                frame "ENL1" {
                  n364 = call "BRig_RT__Case_Exp__State_ENL.vi"("input_dataCurrent"=w1463, "input_dataTrial"=w1453, "input_arrTrig"=w1457, "input_state"=w1456, "I_lick"=w1455) -> ("output_l2_laserOn"=w1458:bool, "output_l2_laserEvent"=w1459:bool, "output_l1_laserOn"=w1460:bool, "output_state"=w1454:T2, "output_l1_laserEvent"=w1461:bool, "output_dataCurrent"=w1462:u16[], "output_dataTrial"=w1452:u16[][])  [unwired: 8 in]
                }
                frame "ENL1Penalty_pre" {
                  n365 = call "BRig_dataCurrent_c_generic.vi"() -> ("output_count_generic"=w1479:i32)  [unwired: 11 in]
                  n366 = call "BRig_dataCurrent_T_generic.vi"() -> ("output_T_generic"=w1477:i32)  [unwired: 11 in]
                  n367 = call "BRig_dataExp_T_ENLPenalty.vi"() -> ("output_ENL_penalty"=w1472:i32)  [unwired: 11 in]
                  n368 = Index Array(array=w1473, index=w1472) -> (element=w1476:u16)
                  n369 = Replace Array Subset(array=w1474, new element #1=u16 0 ("new element/subarray"), index #1=w1479, new element #2=w1476, index #2=w1477) -> (w1475:u16[])
                }
                frame "ENL1Penalty" {
                  n370 = call "BRig_RT__Case_Exp__generic__incrementCountTilThreshold.vi"("input_dataCurrent"=w1482) -> ("output_dataCurrent"=w1481:u16[], "output_underThreshold"=w1480:bool)  [unwired: 9 in]
                  n371 = Select(t=w1485, s=w1480, f=myRIO_BRig_RT__Case_Exp_stateList."ENL1_pre" ("Enum")) -> (s? t:f=w1483:T2)
                }
                frame "Cue1_pre" {
                  n372 = call "BRig_RT__Case_Exp__State_CuePre.vi"("input_dataCurrent"=w1499, "input_dataTrial"=w1495, "input_I_lick"=w1498, "input_dataExp"=w1496, "input_arrTrig"=w1492) -> ("output_state"=w1497:T2, "output_arrTrig"=w1491:bool[], "output_dataCurrent"=w1493:u16[], "output_dataTrial"=w1494:u16[][])  [unwired: 11 in]
                }
                frame "Cue1" {
                  n373 = call "BRig_RT__Case_Exp__State_Cue.vi"("input_dataCurrent"=w1519, "input_dataTrial"=w1507, "input_arrTrig"=w1515, "input_state"=w1517, "I_lick"=w1518) -> ("output_l2_laserOn"=w1511:bool, "output_l2_laserEvent"=w1512:bool, "output_SelectionState"=w1510:bool, "output_l1_laserOn"=w1513:bool, "output_state"=w1516:T2, "output_l1_laserEvent"=w1514:bool, "output_dataCurrent"=w1502:u16[], "output_dataTrial"=w1506:u16[][], "output_CueLed"=w1505:bool, "output_Audio_L"=w1504:bool, "output_Audio_R"=w1503:bool)  [unwired: 4 in]
                  n374 = case shown="True" w1510 {
                    selector: w1510 -> [_ w1525]
                    tunnel: w1509 -> [_ w1524]
                    tunnel: w1508 -> [_ w1523]
                    frame False {
                    }
                    frame True {
                      n375 = xnode "Read/Write Control"("FPGA VI Reference In"=w1523, "error in"=w1524, "SelectionState"=w1525) -> ("error out"=w1526:errorcluster)  [unwired: 1 out]
                      n376 = local write "error out"(w1526) -> ()
                    }
                  }
                }
                frame "Cue1Penalty_pre" {
                  n377 = call "BRig_dataCurrent_c_generic.vi"() -> ("output_count_generic"=w1539:i32)  [unwired: 11 in]
                  n378 = call "BRig_dataCurrent_T_generic.vi"() -> ("output_T_generic"=w1537:i32)  [unwired: 11 in]
                  n379 = call "BRig_dataExp_T_CuePenalty.vi"() -> ("output_T_CuePenalty"=w1528:i32)  [unwired: 11 in]
                  n380 = Index Array(array=w1529, index=w1528) -> (element=w1527:u16)
                  n381 = Replace Array Subset(array=w1536, new element #1=u16 0 ("new element/subarray"), index #1=w1539, new element #2=w1527, index #2=w1537) -> (w1535:u16[])
                }
                frame "Cue1Penalty" {
                  n382 = call "BRig_RT__Case_Exp__generic__incrementCountTilThreshold.vi"("input_dataCurrent"=w1542) -> ("output_dataCurrent"=w1541:u16[], "output_underThreshold"=w1540:bool)  [unwired: 9 in]
                  n383 = Select(t=w1543, s=w1540, f=myRIO_BRig_RT__Case_Exp_stateList."ENL1_pre" ("Enum")) -> (s? t:f=w1544:T2)
                }
                frame "Selection_pre" {
                  n384 = xnode "Read/Write Control"("FPGA VI Reference In"=w1565, "error in"=w1566) -> ("error out"=w1564:errorcluster, "SelectReward"=w1561, "SelectWrong"=w1562)  [unwired: 1 out]
                  n385 = call "BRig_RT__Case_Exp__State_SelectPre.vi"("input_dataCurrent"=w1563, "input_SelectWrong"=w1562, "input_SelectReward"=w1561, "input_dataExp"=w1559, "input_LickL"=w1552, "input_LickR"=w1551, "input_arrTrig"=w1553) -> ("output_state"=w1560:T2, "output_dataCurrent"=w1558:u16[], "output_l1_laserEvent"=w1557:bool, "output_l1_laserOn"=w1556:bool, "output_l2_laserOn"=w1554:bool, "output_l2_laserEvent"=w1555:bool)  [unwired: 3 in]
                  n386 = local write "error out"(w1564) -> ()
                }
                frame "Selection" {
                  n387 = xnode "Read/Write Control"("FPGA VI Reference In"=w1590, "error in"=w1589) -> ("error out"=w1588:errorcluster, "SelectReward"=w1585, "SelectWrong"=w1586)  [unwired: 1 out]
                  n388 = call "BRig_RT__Case_Exp__State_Selection.vi"("input_state"=w1587, "input_dataCurrent"=w1580, "input_dataTrial"=w1571, "input_dataExp"=w1579, "input_arrTrig"=w1578, "input_FPGA_SelectWrong"=w1586, "input_FPGA_SelectReward"=w1585, "input_LickR"=w1584, "input_LickL"=w1583) -> ("output_LC_Laser_l2"=w1574:bool, "output_LC_Event_l2"=w1575:bool, "output_LC_Laser_l1"=w1576:bool, "output_LC_Event_l1"=w1577:bool, "output_state"=w1582:T2, "output_dataCurrent"=w1581:u16[], "output_dataTrial"=w1570:u16[][], "output_anySelect_L"=w1572:bool, "output_anySelect_R"=w1573:bool)  [unwired: 2 in]
                  n389 = local write "allReward_L"(w1572) -> ()
                  n390 = local write "allReward_R"(w1573) -> ()
                  n391 = local write "error out"(w1588) -> ()
                }
                frame "SelectReward_pre" {
                  n392 = call "BRig_RT__Case_Exp__State_RewardPre.vi"("input_dataCurrent"=w1612, "input_dataBlock"=w1611, "input_dataTrial"=w1602) -> ("output_T_Reward"=w1598:u16, "output_c_nReward_total_R"=w1607:u16, "output_c_nReward_total_L"=w1608:u16, "output_dataCurrent"=w1605:u16[], "output_dataBlock"=w1610:u16[][], "output_c_nReward_total"=w1606:u16, "output_nReward"=w1609:u16, "output_dataTrial"=w1601:u16[][])  [unwired: 5 in]
                  n393 = local read "FPGA_count2ms"() -> (w1597:dbl)
                  n394 = local write "nRewards_Right"(w1607) -> ()
                  n395 = local write "nRewards_Left"(w1608) -> ()
                  n396 = local write "nRewards_cur"(w1609) -> ()
                  n397 = local write "nRewards_total"(w1606) -> ()
                  n398 = To Double Precision Float(number=w1598) -> (double precision float=w1596:dbl)
                  n399 = Multiply(x=w1597, y=w1596) -> (x*y=w1594:dbl)
                  n400 = Round Toward +Infinity(x=w1594) -> (ceil(x): smallest int >= x=w1595:dbl)
                  n401 = call "BRig_RT_comm_tcp_write_RTwrite__RunState_Trial_selResult.vi"("input_dataTrial"=w1601, "iReward_or_iError"=TRUE, "input_dataCurrent"=w1605) -> ("output_strCmd"=w1603:string)  [unwired: 8 in]
                  n402 = To Unsigned Long Integer(number=w1595) -> (unsigned 32bit integer=w1593:u32)
                  n403 = xnode "Read/Write Control"("FPGA VI Reference In"=w1600, "error in"=w1599, "Solenoid_nTotal_L"=w1593, "Solenoid_nTotal_R"=w1593) -> ()  [unwired: 2 out]
                }
                frame "SelectReward" {
                  n404 = call "BRig_dataCurrent_c_generic.vi"() -> ("output_count_generic"=w1622:i32)  [unwired: 11 in]
                  n405 = call "BRig_RT__Case_Exp__State_Reward.vi"("input_dataCurrent"=w1623, "input_state"=w1627, "input_dataExp"=w1625) -> ("output_state"=w1626:T2, "output_dataCurrent"=w1628:u16[], "output__L"=w1620:bool, "output__R"=w1619:bool)  [unwired: 5 in, 4 out]
                  n406 = Index Array(array=w1623, index=w1622) -> (element=w1621:u16)
                  n407 = Equal To 0?(x=w1621) -> (x = 0?=w1618:bool)
                  n408 = And(x=w1620, y=w1618) -> (x .and. y?=w1617:bool)
                  n409 = And(x=w1619, y=w1618) -> (x .and. y?=w1616:bool)
                }
                frame "SelectRewardPost_pre" {
                  n410 = call "BRig_dataExp_T_RewardPost.vi"() -> ("output_T_RewardPost"=w1632:i32)  [unwired: 11 in]
                  n411 = call "BRig_dataCurrent_c_generic.vi"() -> ("output_count_generic"=w1638:i32)  [unwired: 11 in]
                  n412 = call "BRig_dataCurrent_T_generic.vi"() -> ("output_T_generic"=w1637:i32)  [unwired: 11 in]
                  n413 = Index Array(array=w1633, index=w1632) -> (element=w1631:u16)
                  n414 = Replace Array Subset(array=w1635, new element #1=u16 0 ("new element/subarray"), index #1=w1638, new element #2=w1631, index #2=w1637) -> (w1634:u16[])
                }
                frame "SelectRewardPost" {
                  n415 = call "BRig_RT__Case_Exp__generic__incrementCountTilThreshold.vi"("input_dataCurrent"=w1645) -> ("output_dataCurrent"=w1643:u16[], "output_underThreshold"=w1644:bool)  [unwired: 9 in]
                  n416 = Select(t=w1647, s=w1644, f=myRIO_BRig_RT__Case_Exp_stateList."endTrial1" ("Enum")) -> (s? t:f=w1646:T2)
                }
                frame "SelectWrong_pre" {
                  n417 = call "BRig_RT__Case_Exp__State_WrongOrTimeout_Pre__v3.vi"("input_dataCurrent"=w1669, "input_WorTO"=FALSE, "input_dataBlock"=w1667, "input_dataTrial"=w1664, "input_dataExp"=w1665) -> ("output_BTPR"=w1658:bool, "output_T2R"=w1659:bool, "output_T2R_or_BTPR"=w1657:u16, "output_dataCurrent"=w1662:u16[], "output_dataBlock"=w1666:u16[][], "output_dataTrial"=w1661:u16[][], "output_BTPRavg"=w1653:dbl, "output_T2Ravg"=w1654:dbl, "output_R(F)_or_L(T)"=w1655:bool, "output_haveNewAvg"=w1656:bool)  [unwired: 1 in]
                  n418 = case shown="True" w1656 {
                    tunnel: w1655 -> [_ w1674]
                    tunnel: w1654 -> [_ w1673]
                    tunnel: w1653 -> [_ w1672]
                    frame False {
                    }
                    frame True {
                      n419 = case shown="False" w1674 {
                        tunnel: w1673 -> [w1675 w1678]
                        tunnel: w1672 -> [w1676 w1677]
                        frame False {
                          n420 = local write "BTPR_avg_R"(w1676) -> ()
                          n421 = local write "T2R_avg_R"(w1675) -> ()
                        }
                        frame True {
                          n422 = local write "BTPR_avg_L"(w1677) -> ()
                          n423 = local write "T2R_avg_L"(w1678) -> ()
                        }
                      }
                    }
                  }
                  n424 = case shown="True" w1659 {
                    tunnel: w1657 -> [_ w1679]
                    frame False {
                    }
                    frame True {
                      n425 = local write "T2R_block"(w1679) -> ()
                    }
                  }
                  n426 = case shown="True" w1658 {
                    tunnel: w1657 -> [_ w1680]
                    frame False {
                    }
                    frame True {
                      n427 = local write "BTPR_block"(w1680) -> ()
                    }
                  }
                  n428 = call "BRig_RT_comm_tcp_write_RTwrite__RunState_Trial_selResult.vi"("input_dataTrial"=w1661, "iReward_or_iError"=FALSE, "input_dataCurrent"=w1662) -> ("output_strCmd"=w1660:string)  [unwired: 8 in]
                }
                frame "SelectWrong" {
                  n429 = call "BRig_RT__Case_Exp__generic__incrementCountTilThreshold.vi"("input_dataCurrent"=w1683) -> ("output_dataCurrent"=w1681:u16[], "output_underThreshold"=w1682:bool)  [unwired: 9 in]
                  n430 = Select(t=w1685, s=w1682, f=myRIO_BRig_RT__Case_Exp_stateList."endTrial1" ("Enum")) -> (s? t:f=w1684:T2)
                }
                frame "SelectTimeout_pre" {
                  n431 = call "BRig_RT__Case_Exp__State_WrongOrTimeout_Pre__v3.vi"("input_dataCurrent"=w1707, "input_WorTO"=TRUE, "input_dataBlock"=w1706, "input_dataTrial"=w1705, "input_dataExp"=w1702) -> ("output_BTPR"=w1696:bool, "output_T2R"=w1697:bool, "output_T2R_or_BTPR"=w1695:u16, "output_dataCurrent"=w1700:u16[], "output_dataBlock"=w1704:u16[][], "output_dataTrial"=w1699:u16[][], "output_BTPRavg"=w1691:dbl, "output_T2Ravg"=w1692:dbl, "output_R(F)_or_L(T)"=w1693:bool, "output_haveNewAvg"=w1694:bool)  [unwired: 1 in]
                  n432 = xnode "Read/Write Control"("FPGA VI Reference In"=w1711, "error in"=w1710, "SelectionState"=FALSE) -> ("error out"=w1708:errorcluster)  [unwired: 1 out]
                  n433 = case shown="True" w1694 {
                    tunnel: w1693 -> [_ w1716]
                    tunnel: w1692 -> [_ w1715]
                    tunnel: w1691 -> [_ w1714]
                    frame False {
                    }
                    frame True {
                      n434 = case shown="False" w1716 {
                        tunnel: w1715 -> [w1717 w1720]
                        tunnel: w1714 -> [w1718 w1719]
                        frame False {
                          n435 = local write "BTPR_avg_R"(w1718) -> ()
                          n436 = local write "T2R_avg_R"(w1717) -> ()
                        }
                        frame True {
                          n437 = local write "BTPR_avg_L"(w1719) -> ()
                          n438 = local write "T2R_avg_L"(w1720) -> ()
                        }
                      }
                    }
                  }
                  n439 = local write "error out"(w1708) -> ()
                  n440 = call "BRig_RT_comm_tcp_write_RTwrite__RunState_Trial_selResult.vi"("input_dataTrial"=w1699, "iReward_or_iError"=FALSE, "input_dataCurrent"=w1700) -> ("output_strCmd"=w1698:string)  [unwired: 8 in]
                  n441 = case shown="True" w1696 {
                    tunnel: w1695 -> [_ w1722]
                    frame False {
                    }
                    frame True {
                      n442 = local write "BTPR_block"(w1722) -> ()
                    }
                  }
                  n443 = case shown="True" w1697 {
                    tunnel: w1695 -> [_ w1721]
                    frame False {
                    }
                    frame True {
                      n444 = local write "T2R_block"(w1721) -> ()
                    }
                  }
                }
                frame "SelectTimeout" {
                  n445 = call "BRig_RT__Case_Exp__generic__incrementCountTilThreshold.vi"("input_dataCurrent"=w1725) -> ("output_dataCurrent"=w1724:u16[], "output_underThreshold"=w1723:bool)  [unwired: 9 in]
                  n446 = Select(t=w1727, s=w1723, f=myRIO_BRig_RT__Case_Exp_stateList."endTrial1" ("Enum")) -> (s? t:f=w1726:T2)
                }
                frame "endTrial1" {
                  n447 = call "BRig_RT_comm_tcp_write_RTwrite__RunState_Trial_end.vi"("input_dataCurrent"=w1740) -> ("output_strCmd"=w1739:string)  [unwired: 10 in]
                  n448 = call "BRig_RT__Case_Exp__State_endTrial__v2.vi"("input_dataBlock"=w1736, "input_timeStamp_start"=w1741, "input_dataTrial"=w1748, "input_dataCurrent"=w1740) -> ("output_BTPRavg"=w1733:dbl, "output_T2Ravg"=w1734:dbl, "output_dataTrial"=w1747:u16[][], "output_dataCurrent"=w1742:u16[], "output_R(F)_or_L(T)"=w1735:bool, "output_runTime"=→"T_ExpRun_min":dbl)  [unwired: 2 in]
                  n449 = xnode "Read/Write Control"("FPGA VI Reference In"=w1744, "error in"=w1743, "SelectionState"=FALSE) -> ("error out"=w1745:errorcluster)  [unwired: 1 out]
                  n450 = case shown="False" w1735 {
                    tunnel: w1734 -> [w1751 w1754]
                    tunnel: w1733 -> [w1752 w1753]
                    frame False {
                      n451 = local write "BTPR_avg_R"(w1752) -> ()
                      n452 = local write "T2R_avg_R"(w1751) -> ()
                    }
                    frame True {
                      n453 = local write "BTPR_avg_L"(w1753) -> ()
                      n454 = local write "T2R_avg_L"(w1754) -> ()
                    }
                  }
                  n455 = local write "error out"(w1745) -> ()
                }
                frame "endTrial2" {
                  n456 = case shown="True" w1764 {
                    tunnel: [w1772 _] -> w1765
                    tunnel: [w1771 w1774] -> w1760
                    tunnel: w1759 -> [w1769 w1782]
                    tunnel: w1758 -> [w1770 w1780]
                    tunnel: [w1770 w1779] -> w1757
                    tunnel: [w1769 w1781] -> w1756
                    tunnel: w1755 -> [_ w1773]
                    frame False {
                      # "Receive commands"
                      n457 = call "BRig_RT__Case_Exp__UploadClosedLoop__v3.vi"() -> ("all rows"=w1772:i64[][], "output_haveCmd"=w1771:bool)  [unwired: 10 in]
                    }
                    frame True {
                      # "Parse commands and update"
                      n458 = Array Size(array=w1773) -> (size(s)=w1778:i32[])
                      n459 = Index Array(array=w1778, index=0) -> (element=w1776:i32)
                      n460 = Not Equal To 0?(x=w1776) -> (x != 0?=w1775:bool)
                      n461 = case shown="False" w1775 {
                        selector: w1775 -> [w1786 w1788]
                        tunnel: w1782 -> [w1784 w1792]
                        tunnel: [w1784 w1791] -> w1781
                        tunnel: w1780 -> [w1783 w1790]
                        tunnel: [w1783 w1789] -> w1779
                        tunnel: [w1786 w1788] -> w1774
                        tunnel: w1773 -> [_ w1787]
                        frame False {
                          w1785 = TRUE ("input_setValues")
                          # "Update"
                          n462 = call "BRig_RT_panel_cue_v0,90.vi"("input_setValues"=w1785, "input_dataExp"=w1784) -> ()  [unwired: 9 in, 1 out]
                          n463 = call "BRig_RT_panel_ExpStruct_v0,96.vi"("input_setValues"=w1785, "input_dataExp"=w1784) -> ()  [unwired: 9 in, 1 out]
                          n464 = call "BRig_RT_panel_Laser1_v0,90.vi"("input_setValues"=w1785, "input_dataExp"=w1784, "input_dataLC"=w1783) -> ()  [unwired: 7 in, 2 out]
                          n465 = call "BRig_RT_panel_Laser2_v0,90.vi"("input_setValues"=w1785, "input_dataExp"=w1784, "input_dataLC"=w1783) -> ()  [unwired: 7 in, 2 out]
                        }
                        frame True {
                          # "Parse"
                          n466 = call "BRig_RT__Case_Exp__UploadClosedLoop__updateSettings.vi"("input_newSettings"=w1787, "input_dataLC"=w1790, "input_dataExp"=w1792) -> ("output_dataLC"=w1789:u16[], "output_dataExp"=w1791:u16[])  [unwired: 7 in]
                        }
                      }
                    }
                  }
                  n467 = Select(t=myRIO_BRig_RT__Case_Exp_stateList."endTrial2", s=w1760, f=myRIO_BRig_RT__Case_Exp_stateList."endTrial3" ("Enum")) -> (s? t:f=w1761:T2)
                }
                frame "endTrial3" {
                  n468 = call "BRig_RT__Case_Exp__endTrial_checkFreeReward.vi"("input_dataBlock"=w1794, "input_dataExp"=w1803, "input_dataTrial"=w1804, "input_dataCurrent"=w1805) -> ("output_state"=w1795:T2, "output_endBlock"=w1793:bool)  [unwired: 6 in]
                  n469 = local read "STOP_endTrial"() -> (w1802:bool)
                  n470 = local read "STOP_abort"() -> (w1801:bool)
                  n471 = local read "START"() -> (w1799:bool)
                  n472 = Not(x=w1799) -> (.not. x?=w1800:bool)
                  n473 = Compound Arithmetic op=OR(w1802, w1800, w1801, w1793) -> (w1798:bool)
                  n474 = Select(t=myRIO_BRig_RT__Case_Exp_stateList."saveData_dataBlock" ("Enum"), s=w1798, f=w1795) -> (s? t:f=w1796:T2)
                }
                frame "endBlock" {
                  # "Get latest\nlaserSwitch"
                  n475 = call "BRig_dataExp_Loop_c_ExpStruct.vi"() -> ("output_Loop_c_ExpStruct"=w1814:i32)  [unwired: 11 in]
                  n476 = call "BRig_dataExp_LaserSwitch.vi"() -> ("output_LaserSwitch"=w1808:i32)  [unwired: 11 in]
                  n477 = local read "START"() -> (w1834:bool)
                  n478 = local read "STOP_endBlock"() -> (w1830:bool)
                  n479 = local read "STOP_endTrial"() -> (w1832:bool)
                  n480 = local read "STOP_abort"() -> (w1831:bool)
                  n481 = Replace Array Subset(array=w1815, new element=u16 2 ("new element/subarray"), index=w1814) -> (w1812:u16[])
                  n482 = call "BRig_RT_panel_ExpStruct_v0,96.vi"("input_setValues"=FALSE, "input_dataExp"=w1812) -> ("output_dataExp"=w1811:u16[])  [unwired: 9 in]
                  n483 = Index Array(array=w1811, index=w1808) -> (element=w1807:u16)
                  n484 = Not(x=w1834) -> (.not. x?=w1833:bool)
                  n485 = Select(t=myRIO_BRig_RT__Case_Exp_stateList."commUpload_dataTrial" ("Enum"), s=w1820, f=myRIO_BRig_RT__Case_Exp_stateList."initBlock" ("Enum")) -> (s? t:f=w1817:T2)
                  n486 = Replace Array Subset(array=w1810, new element=w1807, index=w1808) -> (w1809:u16[])
                  n487 = Compound Arithmetic op=OR(w1833, w1830, w1832, w1831) -> (w1824:bool)
                  n488 = Select(t=myRIO_BRig_RT__Case_Exp_stateList."endExp" ("Enum"), s=w1824, f=w1817) -> (s? t:f=w1835:T2)
                  n489 = Select(t="<S,E>" ("string"), s=w1824, f="") -> (s? t:f=w1821:string)
                }
                frame "endExp" {
                  n490 = xnode "Read/Write Control"("FPGA VI Reference In"=w1838, "error in"=w1837, "A6_Act"=FALSE) -> ("error out"=w1839:errorcluster)  [unwired: 1 out]
                  n491 = local write "error out"(w1839) -> ()
                }
                frame "commUpload_dataTrial" {
                }
                frame "saveData_dataBlock" {
                  n492 = Increment(x=w1869) -> (x+1=w1867:u16)
                  n493 = Replace Array Subset(array=w1861, new element=u16 2 ("new element/subarray"), index=0) -> (w1855:u16[])
                  n494 = Index Array(array=w1853, index (row)=0) -> (element=w1856:u16[])  [unwired: 1 in]
                  n495 = for {
                    tunnel: w1856 -> [w1879] mode=indexing
                    shift-right: [w1878] -> w1854
                    shift-left: w1855 -> [w1882]
                    i -> [w1881]
                    n496 = Increment(x=w1881) -> (x+1=w1880:i32)
                    n497 = Replace Array Subset(array=w1882, new element=w1879, index=w1880) -> (w1878:u16[])
                  }
                  n498 = RT FIFO Write(0:w1864, 1:w1854, 3:w1863) -> (11:w1866:errorcluster)  [unwired: 2 in, 3 out]
                  n499 = Unbundle By Name(w1866) -> ("code"=w1865:i32)
                  n500 = Greater?(x=w1867, y=u16 3) -> (0:w1875:bool)
                  n501 = Equal To 0?(x=w1865) -> (x = 0?=w1862:bool)
                  n502 = Or(x=w1875, y=w1862) -> (x .or. y?=w1874:bool)
                  n503 = Select(t=myRIO_BRig_RT__Case_Exp_stateList."endBlock" ("Enum"), s=w1874, f=w1870) -> (s? t:f=w1868:T2)
                }
                frame "saveData_dataTrial" {
                  n504 = Increment(x=w1900) -> (x+1=w1899:u16)
                  n505 = Replace Array Subset(array=w1885, new element=u16 1 ("new element/subarray"), index=0) -> (w1889:u16[])
                  n506 = Index Array(array=w1884, index (row)=0) -> (element=w1890:u16[])  [unwired: 1 in]
                  n507 = for {
                    tunnel: w1890 -> [w1909] mode=indexing
                    shift-right: [w1908] -> w1888
                    shift-left: w1889 -> [w1912]
                    i -> [w1911]
                    n508 = Increment(x=w1911) -> (x+1=w1910:i32)
                    n509 = Replace Array Subset(array=w1912, new element=w1909, index=w1910) -> (w1908:u16[])
                  }
                  n510 = RT FIFO Write(0:w1887, 1:w1888, 3:w1886) -> (11:w1895:errorcluster)  [unwired: 2 in, 3 out]
                  n511 = Unbundle By Name(w1895) -> ("code"=w1894:i32)
                  n512 = Equal To 0?(x=w1894) -> (x = 0?=w1883:bool)
                  n513 = Greater?(x=w1899, y=u16 3) -> (0:w1897:bool)
                  n514 = Or(x=w1897, y=w1883) -> (x .or. y?=w1896:bool)
                  n515 = Select(t=myRIO_BRig_RT__Case_Exp_stateList."endTrial2" ("Enum"), s=w1896, f=w1901) -> (s? t:f=w1902:T2)
                }
                frame "dummyState" {
                  n516 = call "BRig_dataCurrent_iTrial.vi"() -> ("output_iTrial"=w1919:i32)  [unwired: 11 in]
                  n517 = Index Array(array=w1920, index=w1919) -> (element=w1918:u16)
                  n518 = Equal?(x=w1918, y=u16 1) -> (x = y?=w1916:bool)
                  n519 = Equal To 0?(x=w1927) -> (x = 0?=w1928:bool)
                  n520 = Select(t=u16 13, s=w1916, f=u16 15) -> (s? t:f=w1913:u16)
                  n521 = Select(t=w1913, s=w1928, f=w1927) -> (s? t:f=w1926:u16)
                  n522 = Decrement(x=w1926) -> (x-1=w1925:u16)
                  n523 = Equal To 0?(x=w1925) -> (x = 0?=w1924:bool)
                  n524 = Select(t=myRIO_BRig_RT__Case_Exp_stateList."initTrial" ("Enum"), s=w1924, f=w1922) -> (s? t:f=w1921:T2)
                }
                frame "dummyState_endBlock" {
                  n525 = call "BRig_dataCurrent_iTrial.vi"() -> ("output_iTrial"=w1943:i32)  [unwired: 11 in]
                  n526 = Index Array(array=w1937, index=w1943) -> (element=w1933:u16)
                  n527 = Equal?(x=w1933, y=u16 1) -> (x = y?=w1941:bool)
                  n528 = Equal To 0?(x=w1934) -> (x = 0?=w1945:bool)
                  n529 = Select(t=u16 1, s=w1941, f=u16 3) -> (s? t:f=w1938:u16)
                  n530 = Select(t=w1938, s=w1945, f=w1934) -> (s? t:f=w1944:u16)
                  n531 = Decrement(x=w1944) -> (x-1=w1935:u16)
                  n532 = Equal To 0?(x=w1935) -> (x = 0?=w1936:bool)
                  n533 = Select(t=myRIO_BRig_RT__Case_Exp_stateList."initBlock" ("Enum"), s=w1936, f=w1947) -> (s? t:f=w1946:T2)
                }
                frame "FreeReward_pre" {
                  w1977 = u16 0 ("new element/subarray")
                  # "Duration = MTrig duration"
                  # "Duration = Reward Time"
                  n534 = call "BRig_dataCurrent_FreeReward_c.vi"() -> ("output_FreeReward_c"=w1978:i32)  [unwired: 11 in]
                  n535 = call "BRig_dataCurrent_iSpout.vi"() -> ("output_iSpout"=w1975:i32)  [unwired: 11 in]
                  n536 = call "BRig_dataTrial_T_Reward.vi"() -> ("output_T_Reward"=w1979:i32)  [unwired: 11 in]
                  n537 = call "BRig_dataCurrent_c_generic.vi"() -> ("output_count_generic"=w1984:i32)  [unwired: 11 in]
                  n538 = call "BRig_dataCurrent_T_generic.vi"() -> ("output_T_generic"=w1983:i32)  [unwired: 11 in]
                  n539 = Index Array(array=w1976, index=w1975) -> (element=w1974:u16)
                  n540 = call "BRig_dataMTrig_Solenoid_T_L.vi"() -> ("output_Solenoid_T_L"=w1973:i32)  [unwired: 11 in]
                  n541 = call "BRig_dataMTrig_Solenoid_T_R.vi"() -> ("output_Solenoid_T_R"=w1972:i32)  [unwired: 11 in]
                  n542 = Equal To 0?(x=w1974) -> (x = 0?=w1954:bool)
                  n543 = local read "FPGA_count2ms"() -> (w1966:dbl)
                  n544 = Select(t=w1973, s=w1954, f=w1972) -> (s? t:f=w1970:i32)
                  n545 = Index Array(array=w1980, index (row)=0 ("disabled index (row)"), index (col)=w1979) -> ()  [unwired: 1 out]
                  n546 = Index Array(array=w1971, index=w1970) -> (element=w1965:u16)
                  n547 = Replace Array Subset(array=w1976, new element #1=w1977, index #1=w1978, new element #2=w1977, index #2=w1984, new element #3=w1965, index #3=w1983) -> (w1982:u16[])
                  n548 = To Double Precision Float(number=w1965) -> (double precision float=w1969:dbl)
                  n549 = call "BRig_dataExp_FreeReward_c_L.vi"() -> ("output_FreeReward_c_L"=w1959:i32)  [unwired: 11 in]
                  n550 = call "BRig_dataExp_FreeReward_c_R.vi"() -> ("output_FreeReward_c_R"=w1960:i32)  [unwired: 11 in]
                  n551 = Multiply(x=w1966, y=w1969) -> (x*y=w1967:dbl)
                  n552 = Select(t=w1959, s=w1954, f=w1960) -> (s? t:f=w1956:i32)
                  n553 = Round Toward +Infinity(x=w1967) -> (ceil(x): smallest int >= x=w1968:dbl)
                  n554 = Index Array(array=w1957, index=w1956) -> (element=w1955:u16)
                  n555 = To Unsigned Long Integer(number=w1968) -> (unsigned 32bit integer=w1962:u32)
                  n556 = xnode "Read/Write Control"("FPGA VI Reference In"=w1964, "error in"=w1963, "Solenoid_nTotal_L"=w1962, "Solenoid_nTotal_R"=w1962) -> ()  [unwired: 2 out]
                  n557 = Increment(x=w1955) -> (x+1=w1953:u16)
                  n558 = case shown="False" w1954 {
                    tunnel: w1953 -> [w1987 w1988]
                    frame True {
                      n559 = local write "FreeReward_c_L"(w1987) -> ()
                    }
                    frame False {
                      n560 = local write "FreeReward_c_R"(w1988) -> ()
                    }
                  }
                  n561 = Replace Array Subset(array=w1957, new element=w1953, index=w1956) -> (w1958:u16[])
                }
                frame "FreeReward" {
                  n562 = call "BRig_dataCurrent_iSpout.vi"() -> ("output_iSpout"=w1999:i32)  [unwired: 11 in]
                  n563 = call "BRig_dataCurrent_c_generic.vi"() -> ("output_count_generic"=w1993:i32)  [unwired: 11 in]
                  n564 = Index Array(array=w2000, index #1=w1999, index #2=w1993) -> (element #1=w1998:u16, element #2=w1992:u16)
                  n565 = Equal To 0?(x=w1998) -> (x = 0?=w1996:bool)
                  n566 = Equal To 0?(x=w1992) -> (x = 0?=w1991:bool)
                  n567 = Not(x=w1996) -> (.not. x?=w1997:bool)
                  n568 = call "BRig_RT__Case_Exp__generic__incrementCountTilThreshold.vi"("input_dataCurrent"=w2000) -> ("output_dataCurrent"=w2001:u16[], "output_underThreshold"=w1990:bool)  [unwired: 9 in]
                  n569 = Select(t=w2004, s=w1990, f=myRIO_BRig_RT__Case_Exp_stateList."FreeRewardPost_pre" ("Enum")) -> (s? t:f=w2002:T2)
                  n570 = And(x=w1990, y=w1991) -> (x .and. y?=w1989:bool)
                  n571 = And(x=w1989, y=w1996) -> (x .and. y?=w1994:bool)
                  n572 = And(x=w1989, y=w1997) -> (x .and. y?=w1995:bool)
                }
                frame "FreeRewardPost" {
                  n573 = call "BRig_RT__Case_Exp__generic__incrementCountTilThreshold.vi"("input_dataCurrent"=w2011) -> ("output_dataCurrent"=w2010:u16[], "output_underThreshold"=w2009:bool)  [unwired: 9 in]
                  n574 = Select(t=w2014, s=w2009, f=myRIO_BRig_RT__Case_Exp_stateList."initTrial" ("Enum")) -> (s? t:f=w2012:T2)
                }
                frame "FreeRewardPost_pre" {
                  n575 = call "BRig_dataExp_T_RewardPost.vi"() -> ("output_T_RewardPost"=w2024:i32)  [unwired: 11 in]
                  n576 = call "BRig_dataCurrent_c_generic.vi"() -> ("output_count_generic"=w2027:i32)  [unwired: 11 in]
                  n577 = call "BRig_dataCurrent_T_generic.vi"() -> ("output_T_generic"=w2026:i32)  [unwired: 11 in]
                  n578 = Index Array(array=w2021, index=w2024) -> (element=w2023:u16)
                  n579 = Replace Array Subset(array=w2022, new element #1=u16 0 ("new element/subarray"), index #1=w2027, new element #2=w2023, index #2=w2026) -> (w2020:u16[])
                }
              }
              n580 = call "BRig_RT_panel_manualTriggering_v0,90.vi"("input_dataMTrig"=w1185) -> ("output_Solenoid_R"=w1196:bool, "output_Solenoid_L"=w1195:bool, "output_dataMTrig"=w1228:u16[], "output_Audio_L"=w1227:bool, "output_Audio_R"=w1226:bool, "output_CueLed"=w1224:bool, "output_Laser_l1"=w1200:bool, "output_Laser_l2"=w1220:bool)  [unwired: 11 in]
              n581 = call "BRig_RT__Case_Exp__comm_tcp__data_other.vi"("input_strState"=w1188, "input_strAccum"=w1189, "input_error"=w1190, "input_hTCP"=w1191, "input_I_connected_TCP"=w1192) -> ("output_strAccum"=w1171:string, "output_error"=w1170:errorcluster, "output_hTCP"=w1172:refnum<k5>, "output_I_connect_TCP"=w1173:bool)  [unwired: 3 in]
              n582 = Or(x="STOP_abort", y=w1212) -> (x .or. y?=w1174:bool)
              n583 = Or(x=w1225, y=w1224) -> (x .or. y?=w1203:bool)
              n584 = local read "Laser1_LED"() -> (w1161:bool)
              n585 = local read "Laser2_LED"() -> (w1160:bool)
              n586 = Or(x=w1227, y=w1242) -> (x .or. y?=w1202:bool)
              n587 = Or(x=w1241, y=w1226) -> (x .or. y?=w1201:bool)
              n588 = Or(x=w1199, y=w1200) -> (x .or. y?=w1219:bool)
              n589 = Or(x=w1223, y=w1220) -> (x .or. y?=w1221:bool)
              n590 = call "BRig_RT__Case_Exp__recordLick.vi"("input_dataLick"=w1211, "input_lick__R"=w1205, "input_lick__L"=w1206, "input_lick"=w1207, "intput_state__trialStart"=w1165, "intput_state__trialEnd"=w1210, "input_dataCurrent"=w1209) -> ("output_dataLick"=w1204:u16[][], "output_dataCurrent"=w1208:u16[])  [unwired: 7 in]
              n591 = xnode "Read/Write Control"("FPGA VI Reference In"=w1240, "error in"=w1239, "L1Led_ON"=w1161, "L2Led_ON"=w1160, "Solenoid_trig_L"=w1194, "Solenoid_trig_R"=w1193, "A3_SL"=w1195, "A1_SR"=w1196, "LC_Event_l1"=w1218, "LC_Laser_l1"=w1219, "LC_Event_l2"=w1222, "LC_Laser_l2"=w1221, "CueLed_Event"=w1203, "audioTrigger_L"=w1202, "audioTrigger_R"=w1201) -> ("FPGA VI Reference Out"=w1246:refnum<k20>, "error out"=w1245:errorcluster, "AnaIn_0"=w1186, "AnaIn_1"=w1187)
              n592 = call "BRig_RT__Case_Exp__recordAnalogInput__PortA__fifo__1value.vi"("input_iOccurence"=w1216, "resetOccurrence"=w1215, "input_dataCurrent"=w1209, "input_iState_start"=w1165, "rt fifo"=w1164, "input_iState_end"=w1210, "input_fifo_error"=w1163, "input_AI1"=w1187, "input_AI0"=w1186) -> ("output_fifo_error"=w1169:errorcluster, "output_iOccurrence"=w1217:u16)  [unwired: 8 in, 1 out]
              n593 = call "BRig_RT_timeLoop_Exp__noStateLimit.vi"("input_error"=w1169, "input_Threshold_reset"="input_Threshold_reset", "input_Threshold"=w1231, "input_timestamp"=w1232, "input_state"=w1165) -> ("output_Threshold"=w1229:bool, "output_duration"=→"tLoop":dbl)  [unwired: 4 in, 1 out]
              "Threshold" <- w1229
              n594 = node-c288() -> ()  [unwired: 1 in, 1 out]
            }
            "stop_TimedLoop" <- w862
            n595 = while {
              tunnel: w804 -> [w930]
              tunnel: w803 -> [w929]
              shift-right: [w924] -> _
              shift-left: 0 ("element") -> [w925]
              shift-right: [w920] -> _
              shift-left: w809 -> [w926]
              tunnel: [w923] -> w806
              tunnel: [w922] -> w805
              tunnel: w802 -> [w919]
              tunnel: w801 -> [w918]
              tunnel: [w917] -> w800
              tunnel: [w916] -> w799
              shift-right: [w914] -> _
              shift-left: FALSE -> [w915]
              stop <- w913 stop-if-true
              # "timed out?"
              n596 = RT FIFO Read(0:w930, 3:w929) -> (8:w923:refnum<k33>, 9:w927:u16, 10:w934:bool, 11:w931:errorcluster)  [unwired: 2 in, 1 out]
              n597 = Unbundle By Name(w931) -> ("code"=w935:i32)
              n598 = Not(x=w934) -> (.not. x?=w933:bool)
              n599 = Equal To 0?(x=w935) -> (x = 0?=w932:bool)
              n600 = And(x=w932, y=w933) -> (x .and. y?=w928:bool)
              n601 = Select(t=w931, s=w932, f=w929) -> (s? t:f=w922:errorcluster)
              n602 = case shown="True" w928 {
                tunnel: w927 -> [_ w966]
                tunnel: w926 -> [w958 w968]
                tunnel: w925 -> [w957 w965]
                tunnel: [w958 w967] -> w920
                tunnel: [w957 w961] -> w924
                tunnel: [_ w959] -> w921
                frame False {
                }
                frame True {
                  n603 = Replace Array Subset(array=w968, new element=w966, index=w965) -> (w967:u16[])
                  n604 = Increment(x=w965) -> (x+1=w963:i32)
                  n605 = Less?(x=w965, y=7 ("dimension size")) -> (x < y?=w960:bool)
                  n606 = Select(t=w963, s=w960, f=0) -> (s? t:f=w961:i32)
                  n607 = Not(x=w960) -> (.not. x?=w959:bool)
                }
              }
              n608 = case shown="True" w921 {
                tunnel: w920 -> [_ w947]
                tunnel: w919 -> [w938 w946]
                tunnel: w918 -> [w937 w945]
                tunnel: [w938 w943] -> w917
                tunnel: [w937 w942] -> w916
                tunnel: w915 -> [w936 w940]
                tunnel: [w936 w939] -> w914
                frame False {
                }
                frame True {
                  n609 = for {
                    N: 8 -> [_]
                    tunnel: w947 -> [w954] mode=indexing
                    tunnel: w946 -> [w956]
                    tunnel: w945 -> [w955]
                    shift-right: [w949] -> w941
                    shift-left: FALSE -> [w953]
                    tunnel: [w952] -> w943
                    tunnel: [w951] -> w942
                    n610 = shared-variable-write(w956, w955, w954) -> (w952:refnum<k21>, w951:errorcluster, w950:bool)  [unwired: 1 in]
                    n611 = Or(x=w953, y=w950) -> (x .or. y?=w949:bool)
                  }
                  n612 = Or(x=w940, y=w941) -> (x .or. y?=w939:bool)
                }
              }
              n613 = local read "stop_TimedLoop"() -> (w913:bool)
            }
            n614 = while {
              shift-right: [w1028] -> _
              shift-left: 0 -> [w1017]
              tunnel: w859 -> [w1035]
              tunnel: w851 -> [w1037]
              shift-right: [w1024] -> _
              shift-left: 0 -> [w1019]
              shift-right: [w1029] -> _
              shift-left: w825 -> [w1036]
              shift-right: [w1025] -> _
              shift-left: w824 -> [w1038]
              shift-right: [w1032] -> w848
              shift-left: w818 -> [w1045]
              shift-right: [w1033] -> w841
              shift-left: w817 -> [w1039]
              tunnel: w821 -> [w1022]
              tunnel: w826 -> [w1021]
              stop <- w1046 stop-if-true
              # "nColumns dataBlock"
              # "nColumns dataTrial"
              # "buffer_dataTrial"
              # "buffer_dataBlock"
              # "buffer_dataTrial"
              # "buffer_dataBlock"
              n615 = local read "stop_TimedLoop"() -> (w1046:bool)
              n616 = Not Equal To 0?(x=w1019) -> (x != 0?=w1020:bool)
              n617 = case shown="True" w1020 {
                tunnel: w1038 -> [w1121 w1124]
                tunnel: w1019 -> [w1122 w1126]
                tunnel: w1037 -> [_ w1135]
                tunnel: [w1122 w1123] -> w1026
                tunnel: [w1121 w1124] -> w1027
                frame False {
                }
                frame True {
                  n618 = Array Subset(array=w1124, length (row)=w1126) -> (w1137:u16[][])  [unwired: 3 in]
                  n619 = call "BRig_dataBlock_iBlock.vi"() -> ("output_iBlock"=w1132:i32)  [unwired: 11 in]
                  n620 = Index Array(array=w1124, index (row)=0, index (col)=w1132) -> (element=w1131:u16)
                  n621 = To Double Precision Float(number=w1137) -> (double precision float=w1136:dbl[][])
                  n622 = Not Equal?(x=u16 1, y=w1131) -> (x != y?=w1129:bool)
                  n623 = call-poly <vilib>:"Write To Spreadsheet File.vi"("delimiter (\\t)"="," ("delimiter (\\t)"), "append to file? (new file:F)"=w1129, "2D data"=w1136, "file path (dialog if empty)"=w1135) -> ("new file path (Not A Path if cancelled)"=w1128:path)  [unwired: 4 in]
                  n624 = call <vilib>:"Is Path and Not Empty.vi"("path"=w1128) -> ("Is Path and Not Empty?"=w1127:bool)  [unwired: 4 in]
                  n625 = Select(t=0, s=w1127, f=w1126) -> (s? t:f=w1123:i32)
                }
              }
              n626 = RT FIFO Read(0:w1045, 3:w1039) -> (8:w1032:refnum<k33>, 9:w1023:u16[], 10:w1043:bool, 11:w1040:errorcluster)  [unwired: 2 in, 1 out]
              n627 = Unbundle By Name(w1040) -> ("code"=w1044:i32)
              n628 = Not(x=w1043) -> (.not. x?=w1042:bool)
              n629 = Equal To 0?(x=w1044) -> (x = 0?=w1041:bool)
              n630 = And(x=w1041, y=w1042) -> (x .and. y?=w1034:bool)
              n631 = Select(t=w1040, s=w1041, f=w1039) -> (s? t:f=w1033:errorcluster)
              n632 = Not Equal To 0?(x=w1017) -> (x != 0?=w1018:bool)
              n633 = case shown="True" w1018 {
                tunnel: w1036 -> [w1104 w1107]
                tunnel: w1017 -> [w1105 w1109]
                tunnel: w1035 -> [_ w1118]
                tunnel: [w1105 w1106] -> w1030
                tunnel: [w1104 w1107] -> w1031
                frame False {
                }
                frame True {
                  n634 = Array Subset(array=w1107, length (row)=w1109) -> (w1120:u16[][])  [unwired: 3 in]
                  n635 = call "BRig_dataTrial_nTrial.vi"() -> ("output_nTrial"=w1115:i32)  [unwired: 11 in]
                  n636 = Index Array(array=w1107, index (row)=0, index (col)=w1115) -> (element=w1114:u16)
                  n637 = To Double Precision Float(number=w1120) -> (double precision float=w1119:dbl[][])
                  n638 = Not Equal?(x=u16 1, y=w1114) -> (x != y?=w1112:bool)
                  n639 = call-poly <vilib>:"Write To Spreadsheet File.vi"("delimiter (\\t)"="," ("delimiter (\\t)"), "append to file? (new file:F)"=w1112, "2D data"=w1119, "file path (dialog if empty)"=w1118) -> ("new file path (Not A Path if cancelled)"=w1111:path)  [unwired: 4 in]
                  n640 = call <vilib>:"Is Path and Not Empty.vi"("path"=w1111) -> ("Is Path and Not Empty?"=w1110:bool)  [unwired: 4 in]
                  n641 = Select(t=0, s=w1110, f=w1109) -> (s? t:f=w1106:i32)
                }
              }
              n642 = case shown="True" w1034 {
                tunnel: w1031 -> [w1051 w1061]
                tunnel: w1030 -> [w1050 w1059]
                tunnel: [w1051 w1060] -> w1029
                tunnel: [w1050 w1058] -> w1028
                tunnel: w1027 -> [w1049 w1057]
                tunnel: w1026 -> [w1048 w1055]
                tunnel: [w1049 w1056] -> w1025
                tunnel: [w1048 w1054] -> w1024
                tunnel: w1023 -> [_ w1064]
                tunnel: w1022 -> [_ w1053]
                tunnel: w1021 -> [_ w1052]
                frame False {
                  n643 = Wait (ms)(milliseconds to wait=u32 10) -> ()  [unwired: 1 out]
                }
                frame True {
                  n644 = Index Array(array=w1064, index=0) -> (element=w1062:u16)
                  n645 = Not Equal To 0?(x=w1062) -> (x != 0?=w1063:bool)
                  n646 = case shown="True" w1063 {
                    tunnel: w1064 -> [_ w1080]
                    tunnel: w1062 -> [_ w1083]
                    tunnel: w1061 -> [w1069 w1073]
                    tunnel: [w1069 w1072] -> w1060
                    tunnel: w1059 -> [w1068 w1071]
                    tunnel: [w1068 w1070] -> w1058
                    tunnel: w1057 -> [w1067 w1077]
                    tunnel: [w1067 w1075] -> w1056
                    tunnel: w1055 -> [w1066 w1076]
                    tunnel: [w1066 w1074] -> w1054
                    tunnel: w1053 -> [_ w1079]
                    tunnel: w1052 -> [_ w1078]
                    frame False {
                    }
                    frame True {
                      n647 = Equal?(x=u16 1 ("y"), y=w1083) -> (x = y?=w1081:bool)
                      n648 = case shown="False" w1081 {
                        tunnel: w1080 -> [w1091 w1103]
                        tunnel: w1079 -> [w1089 _]
                        tunnel: w1078 -> [_ w1098]
                        tunnel: w1077 -> [w1093 w1097]
                        tunnel: w1076 -> [w1092 w1099]
                        tunnel: [w1093 w1096] -> w1075
                        tunnel: [w1092 w1095] -> w1074
                        tunnel: w1073 -> [w1088 w1100]
                        tunnel: [w1086 w1100] -> w1072
                        tunnel: w1071 -> [w1085 w1094]
                        tunnel: [w1084 w1094] -> w1070
                        frame True {
                          n649 = Array Subset(array=w1091, index=1, length=w1089) -> (w1087:u16[])
                          n650 = Increment(x=w1085) -> (x+1=w1084:i32)
                          n651 = Replace Array Subset(array=w1088, new element=w1087, index (row)=w1085) -> (w1086:u16[][])  [unwired: 1 in]
                        }
                        frame False {
                          n652 = Array Subset(array=w1103, index=1, length=w1098) -> (w1101:u16[])
                          n653 = Increment(x=w1099) -> (x+1=w1095:i32)
                          n654 = Replace Array Subset(array=w1097, new element=w1101, index (row)=w1099) -> (w1096:u16[][])  [unwired: 1 in]
                        }
                      }
                    }
                  }
                }
              }
            }
            n655 = node-c288(w911) -> ()  [unwired: 1 out]
            n656 = RT FIFO Delete(0:w848, 2:TRUE ("force destroy? (F)"), 3:w841) -> ()  [unwired: 1 out]
            n657 = RT FIFO Delete(0:w806, 2:TRUE ("force destroy? (F)"), 3:w805) -> ()  [unwired: 1 out]
            n658 = flat-sequence {
              tunnel: w882 -> [w1139]
              tunnel: w881 -> [w1142]
              tunnel: w880 -> [w1141]
              tunnel: w879 -> [w1140]
              tunnel: w878 -> [w1144]
              tunnel: w876 -> [_]
              tunnel: w797 -> [w1146]
              tunnel: w846 -> [w1145]
              tunnel: [w1138] -> w857
              tunnel: w841 -> [_]
              tunnel: w875 -> [w1157]
              tunnel: w874 -> [w1156]
              tunnel: w873 -> [w1155]
              tunnel: [w1154] -> w872
              tunnel: [w1153] -> w871
              tunnel: [w1148] -> w867
              tunnel: w857 -> [w1147]
              frame #0 {
                # "Store"
                n659 = call "BRig_RT__Case_Exp__storeData__endExp__v5__p1.vi"("input_dataCurrent"=w1140, "input_dataLC"=w1145, "input_dataExp"=w1146, "input_dataExp_end"=w1141, "input_dataLC_end"=w1142) -> ("output_True"=w1143:bool)  [unwired: 10 in]
                n660 = call "BRig_RT__Case_Exp__storeData__endExp__v5__p2.vi"("input_dataCurrent"=w1140, "input_dataLick"=w1144, "input_True"=w1143, "input_dataMTrig"=w1139) -> ("output_True"=w1138:bool)  [unwired: 11 in]
              }
              frame #1 {
                # "Send"
                n661 = local read "Data Set Prefix"() -> (w1149:string)
                n662 = call "BRig_RT_comm_webdav_upload_all__v3.vi"("input_I_connected_webdav"=w1155, "input_fileName_prefix"=w1149, "input_hSession"=w1156, "input_error"=w1157, "input_True"=w1147) -> ("output_hSession"=w1153:T4, "error out"=w1154:errorcluster, "output_nFilenames"=w1150:i32, "output_arrFilenames"=w1151:string[], "output_uploaded"=w1152:bool[], "output_strCmd"=w1148:string)  [unwired: 5 in]
                n663 = call "BRig_RT_comm_webdav_upload_all_warnUser.vi"("input_n"=w1150, "input_arrFilenames"=w1151, "input_arrUploaded"=w1152) -> ()  [unwired: 9 in]
              }
            }
            n664 = flat-sequence {
              tunnel: w891 -> [w1158]
              tunnel: [w1158] -> w877
              frame #0 {
                w1159 = FALSE ("START")
                n665 = local write "START"(w1159) -> ()
                n666 = local write "STOP_endTrial"(w1159) -> ()
                n667 = local write "STOP_endBlock"(w1159) -> ()
              }
            }
            n668 = xnode "Read/Write Control"("FPGA VI Reference In"=w908, "error in"=w877, "Counts_Reset"=TRUE, "audioTrigger_L"=w894, "audioFreq_L_kHz"=w892, "audioAmp_L"=w893, "audioTrigger_R"=w894, "audioFreq_R_kHz"=w892, "audioAmp_R"=w893, "A3_SL"=w894, "A1_SR"=w894, "A6_Act"=w894) -> ("FPGA VI Reference Out"=w907:refnum<k20>, "error out"=w876:errorcluster)
            n669 = call "BRig_RT__Case_Exp__comm_tcp__data_other.vi"("input_strState"=w867, "input_strAccum"="" ("f"), "input_error"=w868, "input_hTCP"=w869, "input_I_connected_TCP"=w870) -> ("output_error"=w863:errorcluster, "output_hTCP"=w864:refnum<k5>, "output_I_connect_TCP"=w865:bool)  [unwired: 3 in, 1 out]
          }
        }
        n670 = local read "STOP_abort"() -> (w311:bool)
      }
    }
  }
  n671 = flat-sequence {
    tunnel: w89 -> [w2042]
    tunnel: w88 -> [w2044]
    tunnel: w82 -> [w2043]
    tunnel: [w2043] -> w94
    tunnel: [w2042] -> w93
    tunnel: [w2041] -> w92
    tunnel: w67 -> [w2040]
    tunnel: [w2040] -> w91
    tunnel: w68 -> [w2039]
    tunnel: [w2039] -> w90
    tunnel: w75 -> [w2037]
    tunnel: w74 -> [w2036]
    tunnel: w73 -> [w2035]
    tunnel: w69 -> [w2038]
    tunnel: [w2038] -> w87
    tunnel: w86 -> [_]
    tunnel: [w2037] -> w81
    tunnel: [w2036] -> w80
    tunnel: [w2035] -> w79
    tunnel: w94 -> [w2064]
    tunnel: w93 -> [w2063]
    tunnel: w92 -> [w2062]
    tunnel: [w2061] -> _
    tunnel: w91 -> [w2060]
    tunnel: w90 -> [w2059]
    tunnel: w87 -> [w2058]
    tunnel: w81 -> [w2057]
    tunnel: w80 -> [w2056]
    tunnel: w79 -> [w2055]
    frame #0 {
      # "Stop FPGA\nSend QUIT to Host"
      n672 = case shown="True" w2043 {
        tunnel: w2042 -> [_ w2053]
        tunnel: w2044 -> [w2050 w2052]
        tunnel: [w2050 w2051] -> w2041
        frame False {
        }
        frame True {
          n673 = xnode "Read/Write Control"("FPGA VI Reference In"=w2053, "error in"=w2052, "FPGA_Stop"=TRUE) -> ("error out"=w2051:errorcluster)  [unwired: 1 out]
        }
      }
      n674 = case shown="True" w2037 {
        tunnel: w2036 -> [_ w2049]
        tunnel: w2035 -> [_ w2048]
        frame False {
        }
        frame True {
          w2045 = "<S,Q><S,Q><S,Q><S,Q>" ("input_packet")
          n675 = call "BRig_RT_comm_tcp_write_RTwrite.vi"("input_error"=w2048, "input_packet"=w2045, "input_hTCP"=w2049) -> ("output_error"=w2047:errorcluster, "output_hTCP"=w2046:refnum<k5>)  [unwired: 5 in, 2 out]
          n676 = call "BRig_RT_comm_tcp_write_RTwrite.vi"("input_error"=w2047, "input_packet"=w2045, "input_hTCP"=w2046) -> ()  [unwired: 5 in, 4 out]
        }
      }
    }
    frame #1 {
      # "Disconnect FPGA\nDisconnect comm webdav"
      n677 = case shown="True" w2064 {
        tunnel: w2062 -> [w2069 w2072]
        tunnel: w2063 -> [_ w2071]
        tunnel: [w2069 w2070] -> w2061
        frame False {
        }
        frame True {
          n678 = xnode "Close FPGA VI Reference"("FPGA VI Reference In"=w2071, "error in"=w2072) -> ("error out"=w2073:errorcluster)
          n679 = call <vilib>:"Reset myRIO.vi"("error in (no error)"=w2073) -> ("error out"=w2070:errorcluster)  [unwired: 10 in]
        }
      }
      n680 = case shown="True" w2057 {
        tunnel: w2056 -> [_ w2066]
        tunnel: w2055 -> [_ w2065]
        frame False {
        }
        frame True {
          n681 = TCP Close Connection(connection ID=w2066, error in (no error)=w2065) -> ()  [unwired: 1 in, 2 out]
        }
      }
      n682 = case shown="True" w2060 {
        tunnel: w2059 -> [_ w2068]
        tunnel: w2058 -> [_ w2067]
        frame False {
        }
        frame True {
          n683 = call <vilib>:"Close Session.vi"("session handle"=w2068, "error in (no error)"=w2067) -> ()  [unwired: 13 in, 1 out]
        }
      }
    }
  }
  n684 = Flush Stream(8:w6, 11:w7) -> (0:w8:errorcluster, 3:w9:refnum<k21>)  [unwired: 2 in, 1 out]
  n685 = Destroy Stream Endpoint(8:w8, 11:w9) -> ()  [unwired: 1 out]
